vi "Entrenamiento Fuerza 8.vi"(8 "error in (no error)":errorcluster) -> (0 "error out":errorcluster)   [LabVIEW 2014]
panel:
  in  "E/A":bool
  out "Tiempo Restante":string="15 : 58"
  out "Tiempo Transcurrido":string="04 : 01"
  in  "Reset":bool
  out "Hola":string="4"
  out "Cluster":T1={"Label"="Start", "Cuadriceps"=0, "Isquiotibiales"=0, "Gluteos"=0, "Abdomen"=0, "Lumbares"=0, "Dorsales"=0, "Trapecio"=0, "Pectorales"=35, "Biceps"=87, "Opcional"=0, "Tiempo"=20, "Impulso"=4, "Ruptura"=1, "Frecuencia"=80, "Profundidad"=200, "Ganancia"=0.1, "Master"=54, "Slider"=0}
  out "Master Ind":string="54%"
  in  "Master":bool
  out "Master?":bool
  out "error out 2":errorcluster={"status"=FALSE, "code"=1073676418, "source"="VISA Close in Entrenamiento Fuerza 6.vi"}
  in  "Puerto Serial":refnum<visa-resource-name>="COM25"
  out "Start?":bool
  in  "Start":bool
  in  "Impulso":bool
  in  "Back":bool
  in  "Help":bool
  in  "Slider":i32(slide) scale=0.0..100.0
  out "Horizontal Graduated Bar":i16(slide) scale=0.0..100.0
  in  "Remove Button":bool
  in  "Add Button":bool
  out "Opcional %":string="0%"
  in  "Opcional Bool":bool
  out "Biceps %":string="87%"
  in  "Biceps Bool":bool
  out "Pectorales %":string="35%"
  in  "Pectorales Bool":bool
  out "Trapecio %":string="0%"
  in  "Trapecio Bool":bool
  out "Dorsales %":string="0%"
  in  "Dorsales Bool":bool
  out "Lumbares %":string="0%"
  in  "Lumbares Bool":bool
  out "Abdomen %":string="0%"
  in  "Abdomen Bool":bool
  out "Gluteos %":string="0%"
  in  "Gluteos Bool":bool
  out "Isquiotibiales %":string="0%"
  in  "Isquiotibiales Bool":bool
  out "Cuadríceps %":string="0%"
  in  "Cuadriceps Bool":bool
  out "date/time string":string="26/11/2015 06:09:03 p. m."
  # "Entrenamiento de Fuerza"
  # "Presentación"
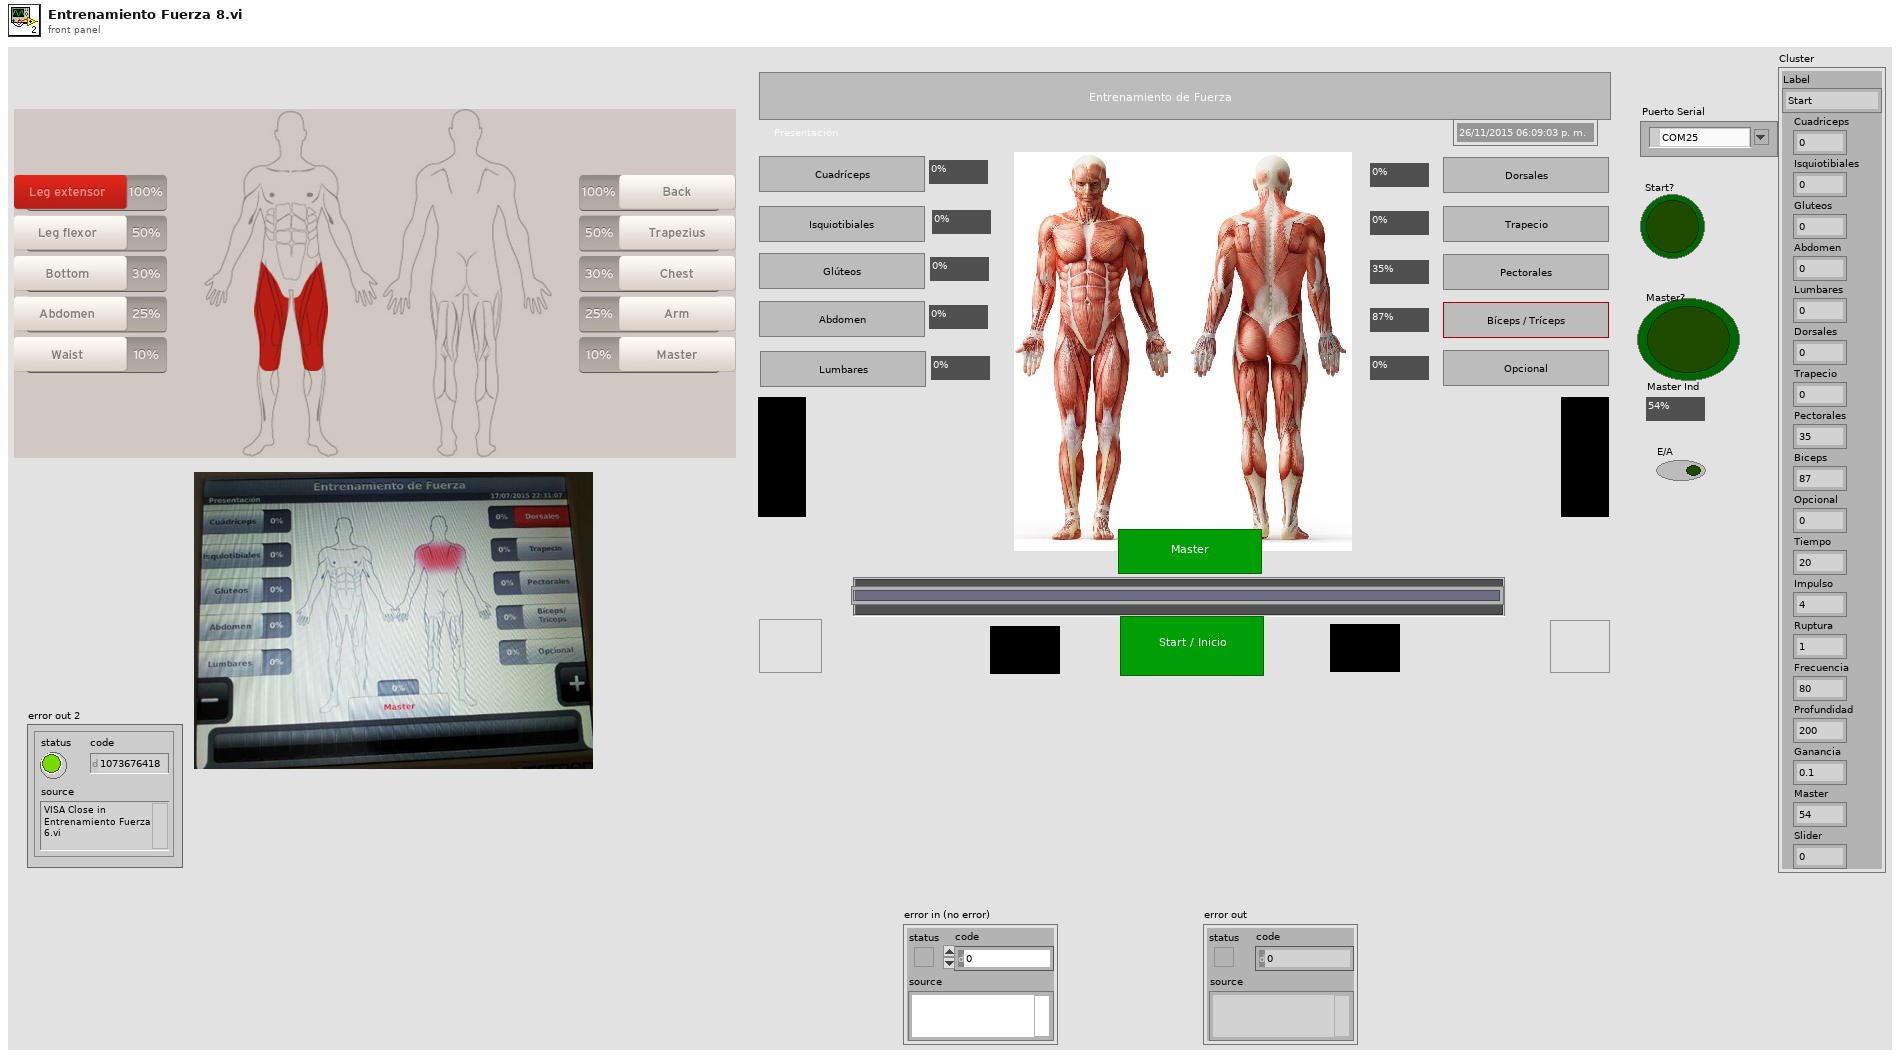
[diagram p1: front panel]
types:
  T1 = cluster{"Label":string, "Cuadriceps":i32, "Isquiotibiales":i32, "Gluteos":i32, "Abdomen":i32, "Lumbares":i32, "Dorsales":i32, "Trapecio":i32, "Pectorales":i32, "Biceps":i32, "Opcional":i32, "Tiempo":i32, "Impulso":i32, "Ruptura":i32, "Frecuencia":i32, "Profundidad":i32, "Ganancia":dbl, "Master":i32, "Slider":i32}
  T2 = cluster{"Label":string, "Cuadriceps":i32, "Isquiotibiales":i32, "Gluteos":i32, "Abdomen":i32, "Lumbares":i32, "Dorsales":i32, "Trapecio":i32, "Pectorales":i32, "Biceps":i32, "Opcional":i32, "Tiempo":i32, "Impulso":i32, "Ruptura":i32, "Frecuencia":i32, "Profundidad":i32, "Ganancia":i32, "Master":i32, "Slider":i32}
  T3 = cluster{u32, "Boolean Text.Text Colors:Text Color":u32}
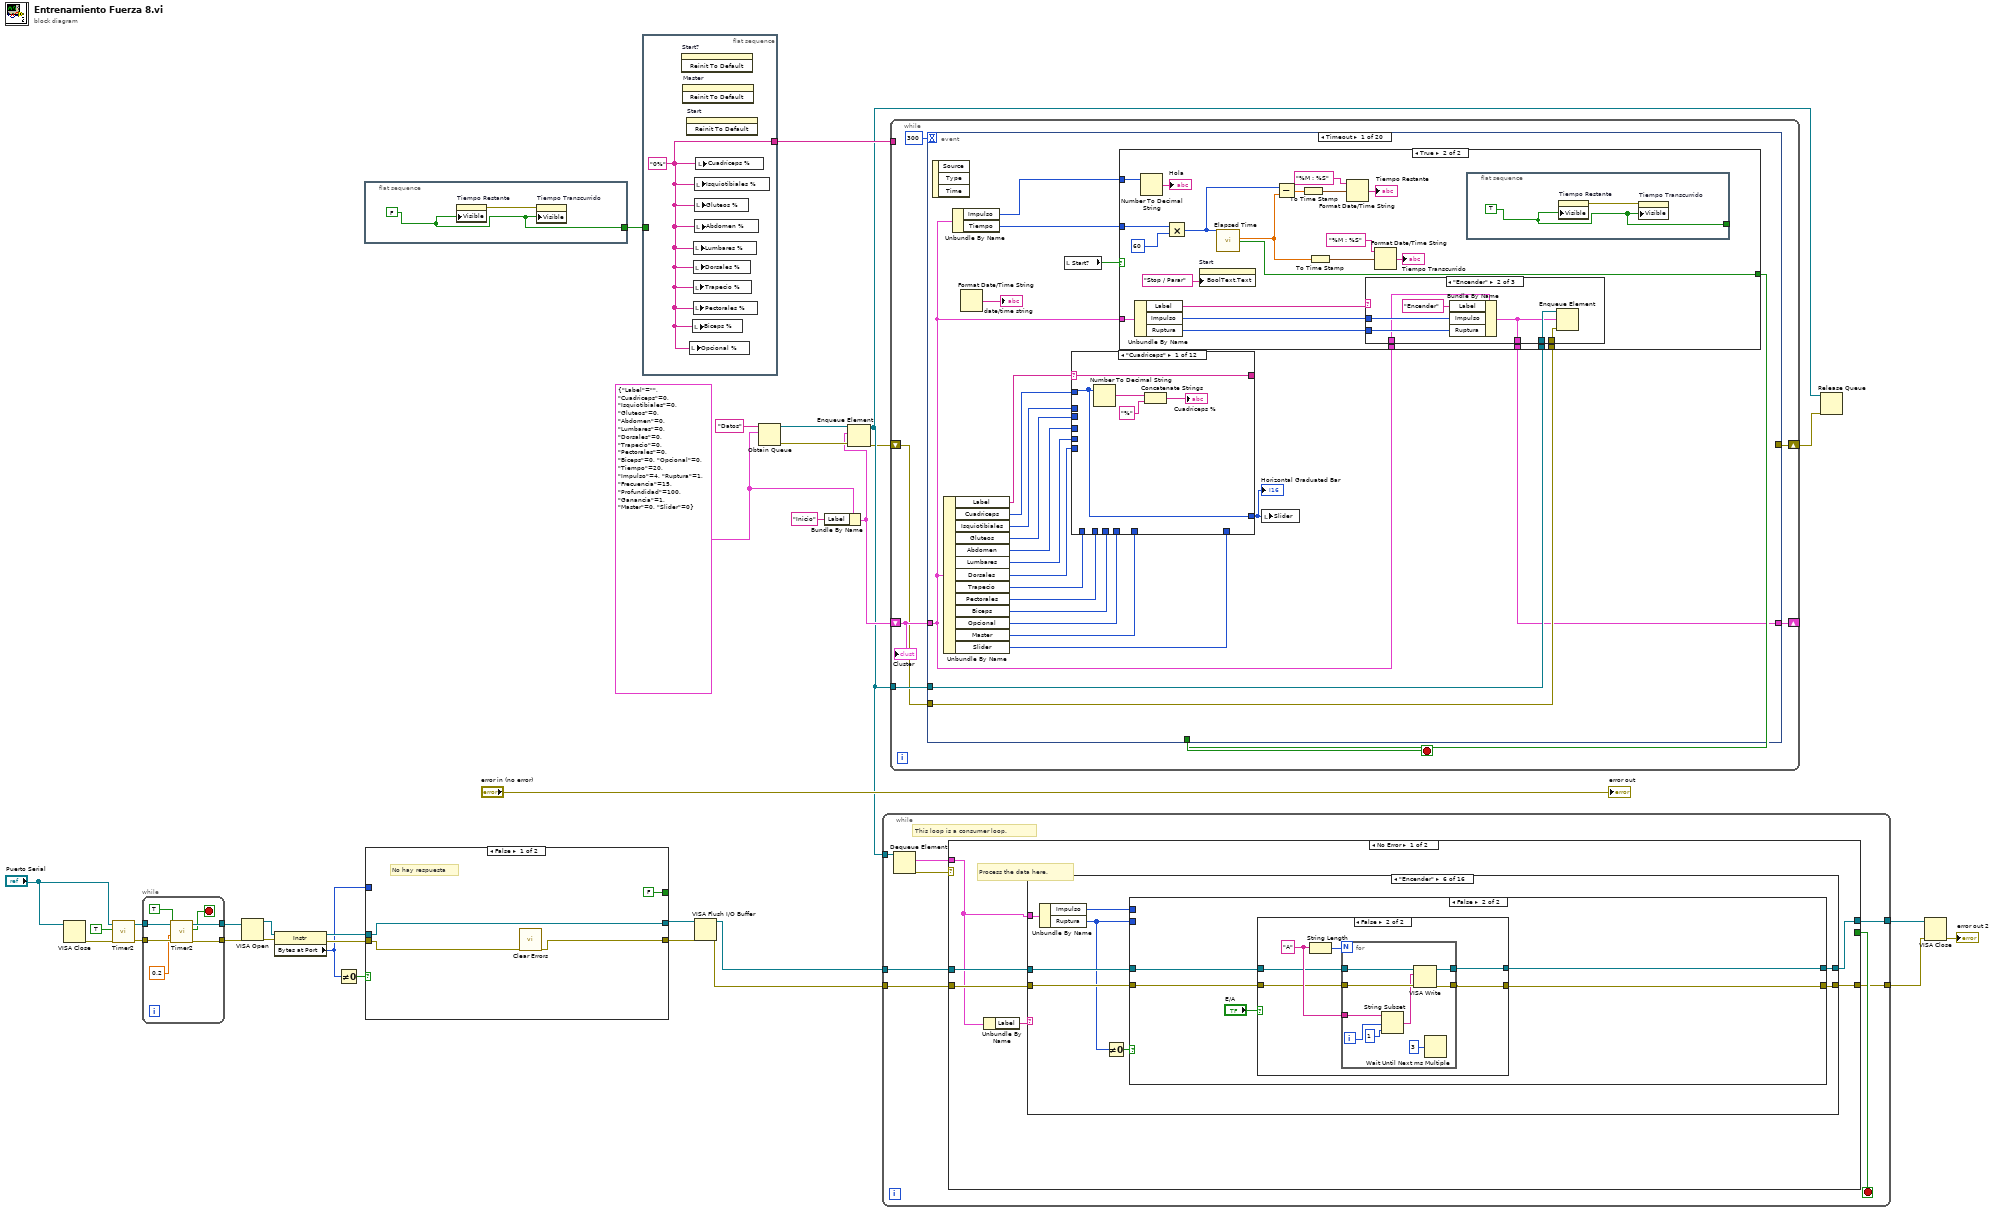
[diagram p0: block diagram]
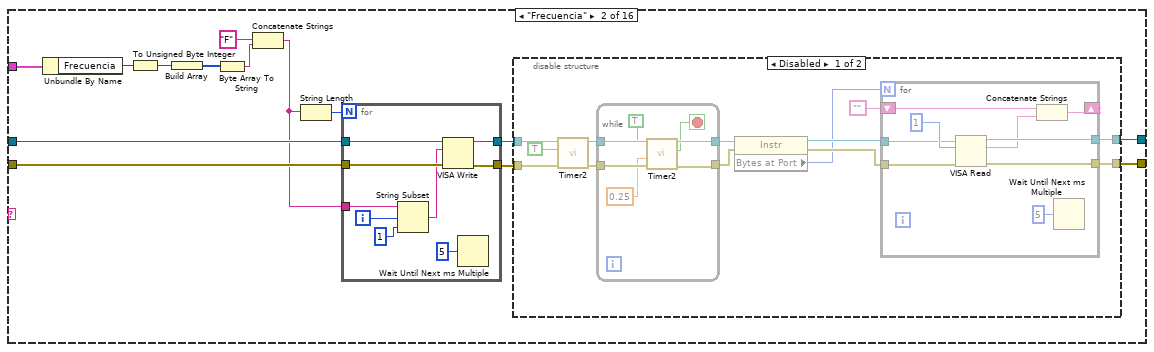
[diagram p3: hidden frame]
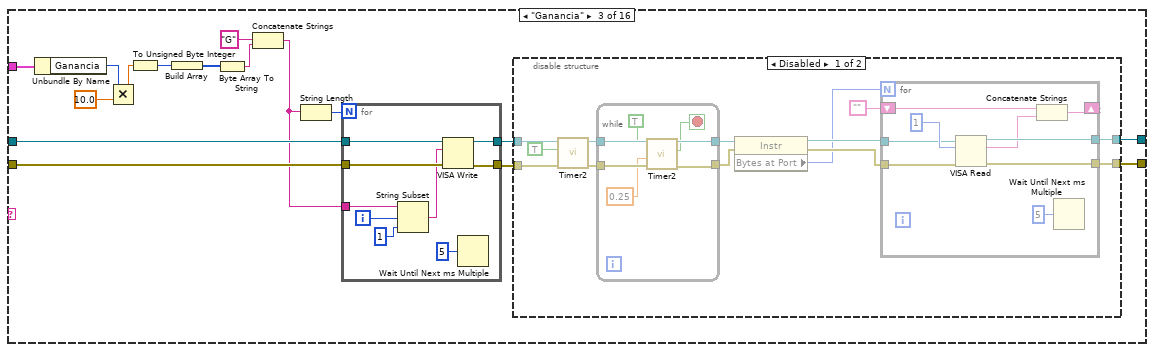
[diagram p5: hidden frame]
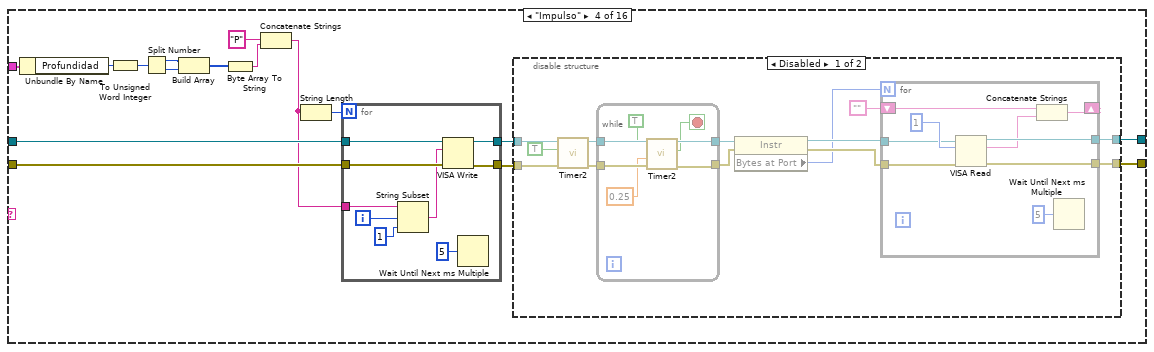
[diagram p7: hidden frame]
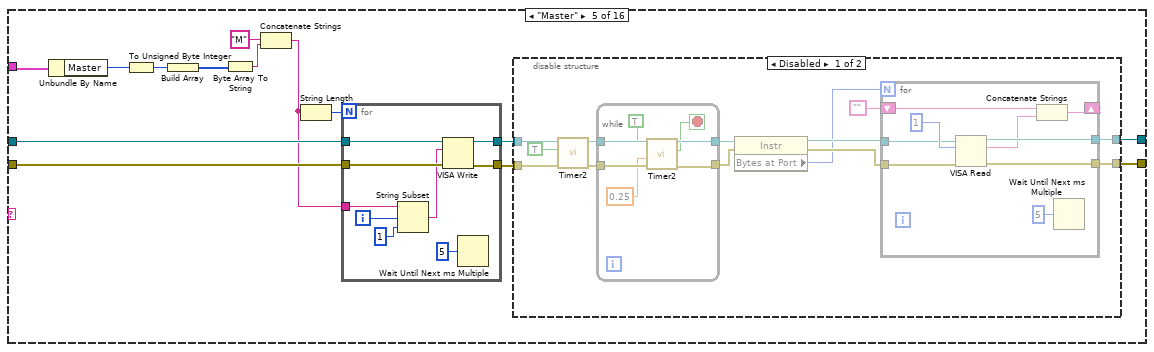
[diagram p9: hidden frame]
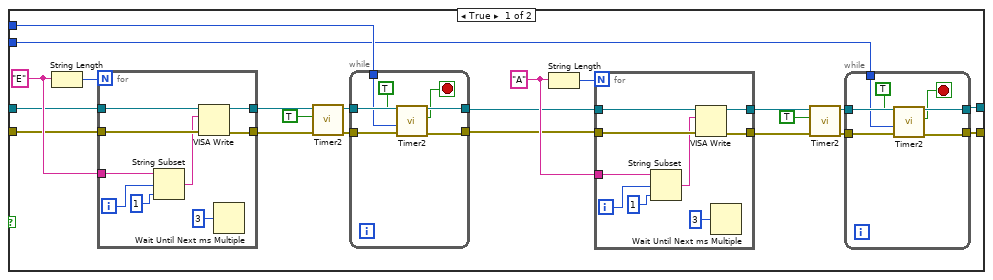
[diagram p11: hidden frame]
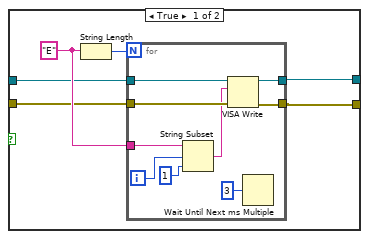
[diagram p12: hidden frame]
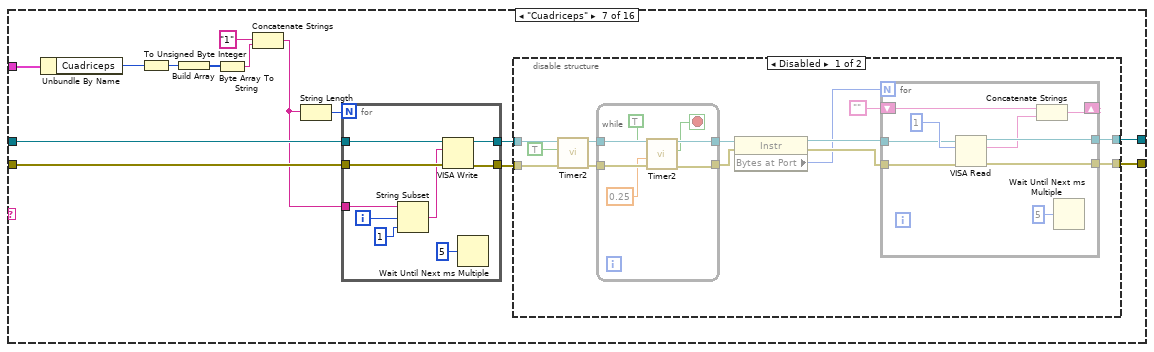
[diagram p13: hidden frame]
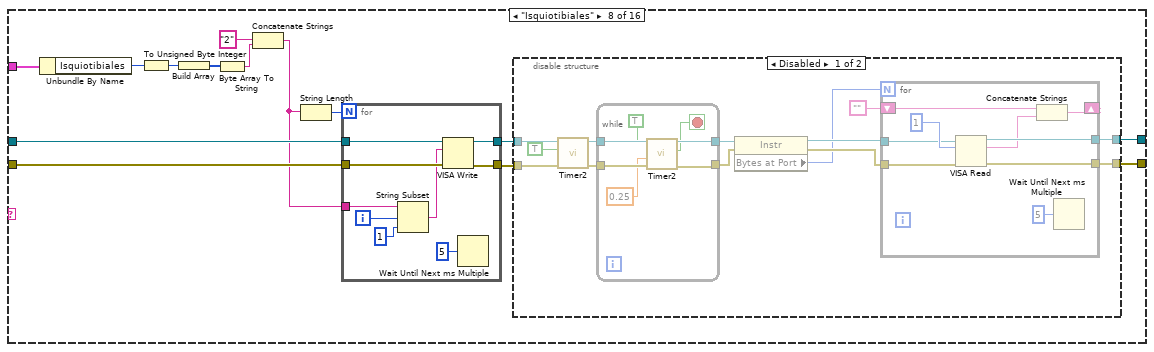
[diagram p15: hidden frame]
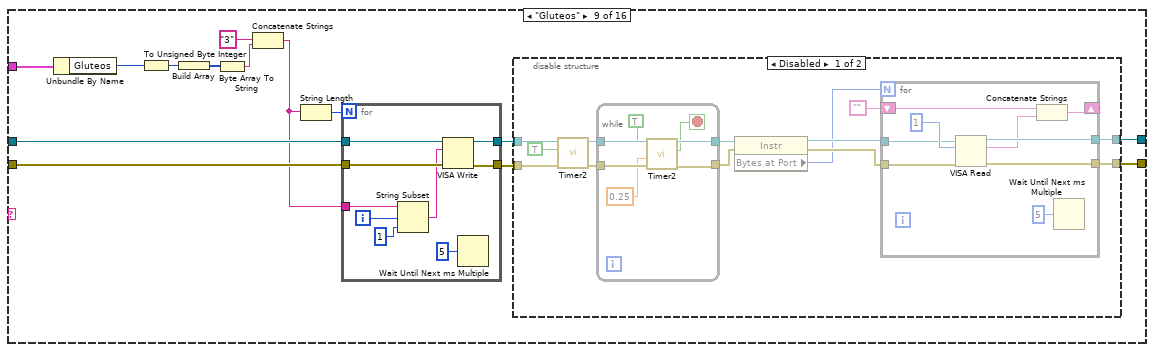
[diagram p17: hidden frame]
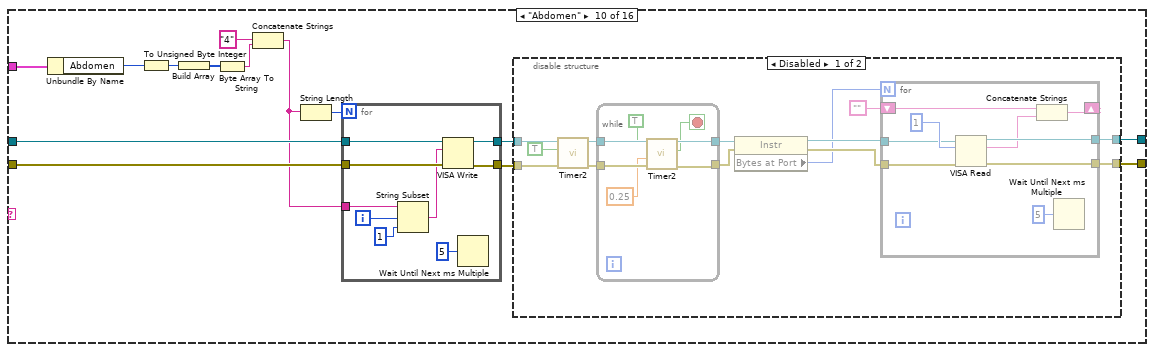
[diagram p19: hidden frame]
diagram:
  w12 = T2 {"Label"="", "Cuadriceps"=0, "Isquiotibiales"=0, "Gluteos"=0, "Abdomen"=0, "Lumbares"=0, "Dorsales"=0, "Trapecio"=0, "Pectorales"=0, "Biceps"=0, "Opcional"=0, "Tiempo"=20, "Impulso"=4, "Ruptura"=1, "Frecuencia"=15, "Profundidad"=100, "Ganancia"=1, "Master"=0, "Slider"=0}
  n1 = VISA Close(VISA resource name="Puerto Serial") -> (error out=w27:errorcluster)  [unwired: 1 in]
  n2 = call "Timer2.vi"("error in (no error)"=w27, "Reset"=TRUE) -> ("error out"=w26:errorcluster)  [unwired: 7 in, 2 out]
  n3 = while {
    tunnel: w26 -> [w36]
    tunnel: "Puerto Serial" -> [w37]
    tunnel: [w37] -> w28
    tunnel: [w35] -> w24
    stop <- w34 stop-if-true
    n4 = call "Timer2.vi"("error in (no error)"=w36, "Time Target (s)"=0.2, "Pause"=TRUE) -> ("error out"=w35:errorcluster, "Time has Elapsed"=w34:bool)  [unwired: 6 in, 1 out]
  }
  n5 = VISA Open(error in (no error)=w24, VISA resource name=w28) -> (VISA resource name=w16:refnum<visa-resource-name>, error out=w17:errorcluster)  [unwired: 3 in]
  n6 = property class="Instr"(reference=w16, error in=w17) -> (reference out=w22:refnum<visa-resource-name>, error out=w23:errorcluster, "Bytes at Port"=w20:u32)
  n7 = Not Equal To 0?(x=w20) -> (x != 0?=w21:bool)
  n8 = flat-sequence {
    tunnel: [w38] -> w1
    frame #0 {
      w38 = FALSE ("Visible")
      n9 = property on="Tiempo Restante" class="Str"("Visible"=w38) -> (error out=w39:errorcluster)  [unwired: 2 in, 1 out]
      n10 = property on="Tiempo Transcurrido" class="Str"(error in=w39, "Visible"=w38) -> ()  [unwired: 1 in, 2 out]
    }
  }
  n11 = case shown="False" w21 {
    tunnel: w23 -> [w41 w51]
    tunnel: w22 -> [w43 w50]
    tunnel: w20 -> [_ w49]
    tunnel: [w43 w47] -> w18
    tunnel: [w40 w46] -> w19
    tunnel: [FALSE w45] -> _
    frame False {
      # "No hay respuesta"
      n12 = call <vilib>:"Clear Errors.vi"("error in (no error)"=w41) -> ("error out"=w40:errorcluster)  [unwired: 5 in, 1 out]
    }
    frame True {
      # "Recibe Datos de Respuesta"
      n13 = for {
        N: w49 -> [_]
        tunnel: w51 -> [w60]
        tunnel: w50 -> [w59]
        shift-right: [w54] -> w44
        shift-left: "" -> [w58]
        tunnel: [w57] -> w46
        tunnel: [w56] -> w47
        n14 = VISA Read(VISA resource name=w59, byte count=u32 1, error in (no error)=w60) -> (VISA resource name out=w56:refnum<visa-resource-name>, read buffer=w53:string, error out=w57:errorcluster)  [unwired: 1 out]
        n15 = Concatenate Strings(w58, w53) -> (w54:string)
        n16 = Wait Until Next ms Multiple(millisecond multiple=u32 1) -> ()  [unwired: 1 out]
      }
      n17 = Equal?(x=w44, y="OK") -> (x = y?=w45:bool)
    }
  }
  n18 = flat-sequence {
    tunnel: [w62] -> w15
    tunnel: w1 -> [_]
    frame #0 {
      w62 = "0%" ("Cuadríceps %")
      n19 = invoke on="Start?" class="Bool (strict)" method="Reinit To Default"() -> ()  [unwired: 3 in, 3 out]
      n20 = invoke on="Master" class="Bool (strict)" method="Reinit To Default"() -> ()  [unwired: 3 in, 3 out]
      n21 = invoke on="Start" class="Bool (strict)" method="Reinit To Default"() -> ()  [unwired: 3 in, 3 out]
      n22 = local write "Opcional %"(w62) -> ()
      n23 = local write "Biceps %"(w62) -> ()
      n24 = local write "Trapecio %"(w62) -> ()
      n25 = local write "Pectorales %"(w62) -> ()
      n26 = local write "Lumbares %"(w62) -> ()
      n27 = local write "Dorsales %"(w62) -> ()
      n28 = local write "Isquiotibiales %"(w62) -> ()
      n29 = local write "Gluteos %"(w62) -> ()
      n30 = local write "Abdomen %"(w62) -> ()
      n31 = local write "Cuadríceps %"(w62) -> ()
    }
  }
  n32 = VISA Flush I/O Buffer(VISA resource name=w18, error in (no error)=w19) -> (VISA resource name out=w7:refnum<visa-resource-name>, error out=w6:errorcluster)  [unwired: 1 in]
  n33 = Obtain Queue(name (unnamed)="Datos", element data type=w12) -> (queue out=w13:refnum<queue>, error out=w14:errorcluster)  [unwired: 3 in, 1 out]
  n34 = Bundle By Name(cluster=w12, "Label"="Inicio") -> (w10:T2)
  n35 = Enqueue Element(queue=w13, element=w10, error in (no error)=w14) -> (queue out=w8:refnum<queue>, error out=w3:errorcluster)  [unwired: 1 in, 1 out]
  n36 = while {
    tunnel: w8 -> [w70]
    tunnel: w7 -> [w66]
    tunnel: w6 -> [w65]
    tunnel: [w64] -> w5
    tunnel: [w63] -> w4
    stop <- w67 stop-if-true
    # "This loop is a consumer loop."
    n37 = Dequeue Element(queue=w70) -> (element=w68:T2, error out=w69:errorcluster)  [unwired: 2 in, 2 out]
    n38 = case shown="No Error" w69 {
      tunnel: w68 -> [w71 _]
      tunnel: [_ TRUE] -> w67
      tunnel: w66 -> [w76 w904]
      tunnel: w65 -> [w75 w905]
      tunnel: [w74 w904] -> w64
      tunnel: [w73 w905] -> w63
      frame No Error {
        # "Process the data here."
        n39 = Unbundle By Name(w71) -> ("Label"=w72:string)
        n40 = case shown="\"Encender\"" w72 {
          tunnel: w76 -> [w77 w92 w146 w200 w252 w295 w397 w449 w501 w553 w605 w657 w709 w761 w813 w865]
          tunnel: w75 -> [w78 w91 w145 w199 w251 w294 w396 w448 w500 w552 w604 w656 w708 w760 w812 w864]
          tunnel: [w78 w90 w144 w198 w250 w297 w395 w447 w499 w551 w603 w655 w707 w759 w811 w863] -> w73
          tunnel: [w77 w89 w143 w197 w249 w296 w394 w446 w498 w550 w602 w654 w706 w758 w810 w862] -> w74
          tunnel: w71 -> [_ w81 w136 w190 w239 w298 w386 w438 w490 w542 w594 w646 w698 w750 w802 w854]
          frame "Inicio", Default {
          }
          frame "Frecuencia" {
            n41 = Unbundle By Name(w81) -> ("Frecuencia"=w82:i32)
            n42 = To Unsigned Byte Integer(number=w82) -> (unsigned 8bit integer=w80:u8)
            n43 = Build Array(w80) -> (w79:u8[])
            n44 = Byte Array To String(unsigned byte array=w79) -> (string=w84:string)
            n45 = Concatenate Strings("F", w84) -> (w83:string)
            n46 = String Length(string=w83) -> (length=w88:i32)
            n47 = for {
              N: w88 -> [_]
              tunnel: w91 -> [w130]
              tunnel: w92 -> [w129]
              tunnel: w83 -> [w126]
              tunnel: [w123] -> w86
              tunnel: [w122] -> w87
              i -> [w124]
              n48 = String Subset(string=w126, offset (0)=w124, length (rest)=1 ("length (rest)")) -> (substring=w127:string)
              n49 = VISA Write(VISA resource name=w129, write buffer=w127, error in (no error)=w130) -> (VISA resource name out=w122:refnum<visa-resource-name>, error out=w123:errorcluster)  [unwired: 1 out]
              n50 = Wait Until Next ms Multiple(millisecond multiple=u32 5) -> ()  [unwired: 1 out]
            }
            n51 = disable-structure shown="Disabled" {
              disable-tunnel: [w104 w120] -> w90
              disable-tunnel: [w103 w121] -> w89
              disable-tunnel: w87 -> [w98 w121]
              disable-tunnel: w86 -> [w94 w120]
              frame Disabled {
                n52 = call "Timer2.vi"("error in (no error)"=w94, "Reset"=TRUE) -> ("error out"=w93:errorcluster)  [unwired: 7 in, 2 out]
                n53 = while {
                  tunnel: w98 -> [w110]
                  tunnel: [w110] -> w97
                  tunnel: [w108] -> w96
                  tunnel: w93 -> [w109]
                  stop <- w107 stop-if-true
                  n54 = call "Timer2.vi"("error in (no error)"=w109, "Time Target (s)"=0.25, "Pause"=TRUE) -> ("error out"=w108:errorcluster, "Time has Elapsed"=w107:bool)  [unwired: 6 in, 1 out]
                }
                n55 = property class="Instr"(reference=w97, error in=w96) -> (reference out=w101:refnum<visa-resource-name>, error out=w100:errorcluster, "Bytes at Port"=w99:u32)
                n56 = for {
                  N: w99 -> [_]
                  tunnel: w100 -> [w118]
                  tunnel: w101 -> [w117]
                  shift-right: [w112] -> _
                  shift-left: "" -> [w116]
                  tunnel: [w115] -> w104
                  tunnel: [w114] -> w103
                  n57 = VISA Read(VISA resource name=w117, byte count=u32 1, error in (no error)=w118) -> (VISA resource name out=w114:refnum<visa-resource-name>, read buffer=w111:string, error out=w115:errorcluster)  [unwired: 1 out]
                  n58 = Concatenate Strings(w116, w111) -> (w112:string)
                  n59 = Wait Until Next ms Multiple(millisecond multiple=u32 5) -> ()  [unwired: 1 out]
                }
              }
              frame Enabled {
              }
            }
          }
          frame "Ganancia" {
            n60 = Unbundle By Name(w136) -> ("Ganancia"=w132:i32)
            n61 = Multiply(x=w132, y=10.0) -> (x*y=w133:dbl)
            n62 = To Unsigned Byte Integer(number=w133) -> (unsigned 8bit integer=w135:u8)
            n63 = Build Array(w135) -> (w134:u8[])
            n64 = Byte Array To String(unsigned byte array=w134) -> (string=w138:string)
            n65 = Concatenate Strings("G", w138) -> (w137:string)
            n66 = String Length(string=w137) -> (length=w142:i32)
            n67 = for {
              N: w142 -> [_]
              tunnel: w145 -> [w184]
              tunnel: w146 -> [w183]
              tunnel: w137 -> [w180]
              tunnel: [w177] -> w140
              tunnel: [w176] -> w141
              i -> [w178]
              n68 = String Subset(string=w180, offset (0)=w178, length (rest)=1 ("length (rest)")) -> (substring=w181:string)
              n69 = VISA Write(VISA resource name=w183, write buffer=w181, error in (no error)=w184) -> (VISA resource name out=w176:refnum<visa-resource-name>, error out=w177:errorcluster)  [unwired: 1 out]
              n70 = Wait Until Next ms Multiple(millisecond multiple=u32 5) -> ()  [unwired: 1 out]
            }
            n71 = disable-structure shown="Disabled" {
              disable-tunnel: [w158 w174] -> w144
              disable-tunnel: [w157 w175] -> w143
              disable-tunnel: w141 -> [w152 w175]
              disable-tunnel: w140 -> [w148 w174]
              frame Disabled {
                n72 = call "Timer2.vi"("error in (no error)"=w148, "Reset"=TRUE) -> ("error out"=w147:errorcluster)  [unwired: 7 in, 2 out]
                n73 = while {
                  tunnel: w152 -> [w164]
                  tunnel: [w164] -> w151
                  tunnel: [w162] -> w150
                  tunnel: w147 -> [w163]
                  stop <- w161 stop-if-true
                  n74 = call "Timer2.vi"("error in (no error)"=w163, "Time Target (s)"=0.25, "Pause"=TRUE) -> ("error out"=w162:errorcluster, "Time has Elapsed"=w161:bool)  [unwired: 6 in, 1 out]
                }
                n75 = property class="Instr"(reference=w151, error in=w150) -> (reference out=w155:refnum<visa-resource-name>, error out=w154:errorcluster, "Bytes at Port"=w153:u32)
                n76 = for {
                  N: w153 -> [_]
                  tunnel: w154 -> [w172]
                  tunnel: w155 -> [w171]
                  shift-right: [w166] -> _
                  shift-left: "" -> [w170]
                  tunnel: [w169] -> w158
                  tunnel: [w168] -> w157
                  n77 = VISA Read(VISA resource name=w171, byte count=u32 1, error in (no error)=w172) -> (VISA resource name out=w168:refnum<visa-resource-name>, read buffer=w165:string, error out=w169:errorcluster)  [unwired: 1 out]
                  n78 = Concatenate Strings(w170, w165) -> (w166:string)
                  n79 = Wait Until Next ms Multiple(millisecond multiple=u32 5) -> ()  [unwired: 1 out]
                }
              }
              frame Enabled {
              }
            }
          }
          frame "Impulso" {
            n80 = Unbundle By Name(w190) -> ("Profundidad"=w187:i32)
            n81 = To Unsigned Word Integer(number=w187) -> (unsigned 16bit integer=w186:u16)
            n82 = Split Number(x=w186) -> (hi(x)=w189:u8, lo(x)=w188:u8)
            n83 = Build Array(w189, w188) -> (w185:u8[])
            n84 = Byte Array To String(unsigned byte array=w185) -> (string=w192:string)
            n85 = Concatenate Strings("P", w192) -> (w191:string)
            n86 = String Length(string=w191) -> (length=w196:i32)
            n87 = for {
              N: w196 -> [_]
              tunnel: w199 -> [w238]
              tunnel: w200 -> [w237]
              tunnel: w191 -> [w234]
              tunnel: [w231] -> w194
              tunnel: [w230] -> w195
              i -> [w232]
              n88 = String Subset(string=w234, offset (0)=w232, length (rest)=1 ("length (rest)")) -> (substring=w235:string)
              n89 = VISA Write(VISA resource name=w237, write buffer=w235, error in (no error)=w238) -> (VISA resource name out=w230:refnum<visa-resource-name>, error out=w231:errorcluster)  [unwired: 1 out]
              n90 = Wait Until Next ms Multiple(millisecond multiple=u32 5) -> ()  [unwired: 1 out]
            }
            n91 = disable-structure shown="Disabled" {
              disable-tunnel: [w212 w228] -> w198
              disable-tunnel: [w211 w229] -> w197
              disable-tunnel: w195 -> [w206 w229]
              disable-tunnel: w194 -> [w202 w228]
              frame Disabled {
                n92 = call "Timer2.vi"("error in (no error)"=w202, "Reset"=TRUE) -> ("error out"=w201:errorcluster)  [unwired: 7 in, 2 out]
                n93 = while {
                  tunnel: w206 -> [w218]
                  tunnel: [w218] -> w205
                  tunnel: [w216] -> w204
                  tunnel: w201 -> [w217]
                  stop <- w215 stop-if-true
                  n94 = call "Timer2.vi"("error in (no error)"=w217, "Time Target (s)"=0.25, "Pause"=TRUE) -> ("error out"=w216:errorcluster, "Time has Elapsed"=w215:bool)  [unwired: 6 in, 1 out]
                }
                n95 = property class="Instr"(reference=w205, error in=w204) -> (reference out=w209:refnum<visa-resource-name>, error out=w208:errorcluster, "Bytes at Port"=w207:u32)
                n96 = for {
                  N: w207 -> [_]
                  tunnel: w208 -> [w226]
                  tunnel: w209 -> [w225]
                  shift-right: [w220] -> _
                  shift-left: "" -> [w224]
                  tunnel: [w223] -> w212
                  tunnel: [w222] -> w211
                  n97 = VISA Read(VISA resource name=w225, byte count=u32 1, error in (no error)=w226) -> (VISA resource name out=w222:refnum<visa-resource-name>, read buffer=w219:string, error out=w223:errorcluster)  [unwired: 1 out]
                  n98 = Concatenate Strings(w224, w219) -> (w220:string)
                  n99 = Wait Until Next ms Multiple(millisecond multiple=u32 5) -> ()  [unwired: 1 out]
                }
              }
              frame Enabled {
              }
            }
          }
          frame "Master" {
            n100 = Unbundle By Name(w239) -> ("Master"=w242:i32)
            n101 = To Unsigned Byte Integer(number=w242) -> (unsigned 8bit integer=w241:u8)
            n102 = Build Array(w241) -> (w240:u8[])
            n103 = Byte Array To String(unsigned byte array=w240) -> (string=w244:string)
            n104 = Concatenate Strings("M", w244) -> (w243:string)
            n105 = String Length(string=w243) -> (length=w248:i32)
            n106 = for {
              N: w248 -> [_]
              tunnel: w251 -> [w290]
              tunnel: w252 -> [w289]
              tunnel: w243 -> [w286]
              tunnel: [w283] -> w246
              tunnel: [w282] -> w247
              i -> [w284]
              n107 = String Subset(string=w286, offset (0)=w284, length (rest)=1 ("length (rest)")) -> (substring=w287:string)
              n108 = VISA Write(VISA resource name=w289, write buffer=w287, error in (no error)=w290) -> (VISA resource name out=w282:refnum<visa-resource-name>, error out=w283:errorcluster)  [unwired: 1 out]
              n109 = Wait Until Next ms Multiple(millisecond multiple=u32 5) -> ()  [unwired: 1 out]
            }
            n110 = disable-structure shown="Disabled" {
              disable-tunnel: [w264 w280] -> w250
              disable-tunnel: [w263 w281] -> w249
              disable-tunnel: w247 -> [w258 w281]
              disable-tunnel: w246 -> [w254 w280]
              frame Disabled {
                n111 = call "Timer2.vi"("error in (no error)"=w254, "Reset"=TRUE) -> ("error out"=w253:errorcluster)  [unwired: 7 in, 2 out]
                n112 = while {
                  tunnel: w258 -> [w270]
                  tunnel: [w270] -> w257
                  tunnel: [w268] -> w256
                  tunnel: w253 -> [w269]
                  stop <- w267 stop-if-true
                  n113 = call "Timer2.vi"("error in (no error)"=w269, "Time Target (s)"=0.25, "Pause"=TRUE) -> ("error out"=w268:errorcluster, "Time has Elapsed"=w267:bool)  [unwired: 6 in, 1 out]
                }
                n114 = property class="Instr"(reference=w257, error in=w256) -> (reference out=w261:refnum<visa-resource-name>, error out=w260:errorcluster, "Bytes at Port"=w259:u32)
                n115 = for {
                  N: w259 -> [_]
                  tunnel: w260 -> [w278]
                  tunnel: w261 -> [w277]
                  shift-right: [w272] -> _
                  shift-left: "" -> [w276]
                  tunnel: [w275] -> w264
                  tunnel: [w274] -> w263
                  n116 = VISA Read(VISA resource name=w277, byte count=u32 1, error in (no error)=w278) -> (VISA resource name out=w274:refnum<visa-resource-name>, read buffer=w271:string, error out=w275:errorcluster)  [unwired: 1 out]
                  n117 = Concatenate Strings(w276, w271) -> (w272:string)
                  n118 = Wait Until Next ms Multiple(millisecond multiple=u32 5) -> ()  [unwired: 1 out]
                }
              }
              frame Enabled {
              }
            }
          }
          frame "Encender" {
            n119 = Unbundle By Name(w298) -> ("Impulso"=w293:i32, "Ruptura"=w291:i32)
            n120 = Not Equal To 0?(x=w291) -> (x != 0?=w292:bool)
            n121 = case shown="False" w292 {
              tunnel: [w304 w351] -> w297
              tunnel: [w303 w350] -> w296
              tunnel: w295 -> [w302 w353]
              tunnel: w294 -> [w301 w352]
              tunnel: w293 -> [w300 _]
              tunnel: w291 -> [w299 _]
              frame True {
                w309 = "A"
                w315 = "E"
                n122 = String Length(string=w315) -> (length=w318:i32)
                n123 = for {
                  N: w318 -> [_]
                  tunnel: w301 -> [w348]
                  tunnel: w302 -> [w347]
                  tunnel: w315 -> [w344]
                  tunnel: [w341] -> w316
                  tunnel: [w340] -> w317
                  i -> [w342]
                  n124 = String Subset(string=w344, offset (0)=w342, length (rest)=1 ("length (rest)")) -> (substring=w345:string)
                  n125 = VISA Write(VISA resource name=w347, write buffer=w345, error in (no error)=w348) -> (VISA resource name out=w340:refnum<visa-resource-name>, error out=w341:errorcluster)  [unwired: 1 out]
                  n126 = Wait Until Next ms Multiple(millisecond multiple=u32 3) -> ()  [unwired: 1 out]
                }
                n127 = call "Timer2.vi"("error in (no error)"=w316, "Reset"=TRUE) -> ("error out"=w313:errorcluster)  [unwired: 7 in, 2 out]
                n128 = while {
                  tunnel: w317 -> [w339]
                  tunnel: [w339] -> w306
                  tunnel: [w337] -> w305
                  tunnel: w313 -> [w338]
                  tunnel: w300 -> [w334]
                  stop <- w336 stop-if-true
                  n129 = call "Timer2.vi"("error in (no error)"=w338, "Time Target (s)"=w334, "Pause"=TRUE) -> ("error out"=w337:errorcluster, "Time has Elapsed"=w336:bool)  [unwired: 6 in, 1 out]
                }
                n130 = String Length(string=w309) -> (length=w312:i32)
                n131 = for {
                  N: w312 -> [_]
                  tunnel: w305 -> [w333]
                  tunnel: w306 -> [w332]
                  tunnel: w309 -> [w329]
                  tunnel: [w326] -> w310
                  tunnel: [w325] -> w311
                  i -> [w327]
                  n132 = String Subset(string=w329, offset (0)=w327, length (rest)=1 ("length (rest)")) -> (substring=w330:string)
                  n133 = VISA Write(VISA resource name=w332, write buffer=w330, error in (no error)=w333) -> (VISA resource name out=w325:refnum<visa-resource-name>, error out=w326:errorcluster)  [unwired: 1 out]
                  n134 = Wait Until Next ms Multiple(millisecond multiple=u32 3) -> ()  [unwired: 1 out]
                }
                n135 = call "Timer2.vi"("error in (no error)"=w310, "Reset"=TRUE) -> ("error out"=w307:errorcluster)  [unwired: 7 in, 2 out]
                n136 = while {
                  tunnel: w311 -> [w324]
                  tunnel: [w324] -> w303
                  tunnel: [w322] -> w304
                  tunnel: w307 -> [w323]
                  tunnel: w299 -> [w319]
                  stop <- w321 stop-if-true
                  n137 = call "Timer2.vi"("error in (no error)"=w323, "Time Target (s)"=w319, "Pause"=TRUE) -> ("error out"=w322:errorcluster, "Time has Elapsed"=w321:bool)  [unwired: 6 in, 1 out]
                }
              }
              frame False {
                n138 = case shown="False" "E/A" {
                  tunnel: w353 -> [w357 w372]
                  tunnel: w352 -> [w356 w371]
                  tunnel: [w355 w370] -> w351
                  tunnel: [w354 w369] -> w350
                  frame True {
                    w358 = "E"
                    n139 = String Length(string=w358) -> (length=w359:i32)
                    n140 = for {
                      N: w359 -> [_]
                      tunnel: w356 -> [w368]
                      tunnel: w357 -> [w367]
                      tunnel: w358 -> [w364]
                      tunnel: [w361] -> w355
                      tunnel: [w360] -> w354
                      i -> [w362]
                      n141 = String Subset(string=w364, offset (0)=w362, length (rest)=1 ("length (rest)")) -> (substring=w365:string)
                      n142 = VISA Write(VISA resource name=w367, write buffer=w365, error in (no error)=w368) -> (VISA resource name out=w360:refnum<visa-resource-name>, error out=w361:errorcluster)  [unwired: 1 out]
                      n143 = Wait Until Next ms Multiple(millisecond multiple=u32 3) -> ()  [unwired: 1 out]
                    }
                  }
                  frame False {
                    w373 = "A"
                    n144 = String Length(string=w373) -> (length=w374:i32)
                    n145 = for {
                      N: w374 -> [_]
                      tunnel: w371 -> [w383]
                      tunnel: w372 -> [w382]
                      tunnel: w373 -> [w379]
                      tunnel: [w376] -> w370
                      tunnel: [w375] -> w369
                      i -> [w377]
                      n146 = String Subset(string=w379, offset (0)=w377, length (rest)=1 ("length (rest)")) -> (substring=w380:string)
                      n147 = VISA Write(VISA resource name=w382, write buffer=w380, error in (no error)=w383) -> (VISA resource name out=w375:refnum<visa-resource-name>, error out=w376:errorcluster)  [unwired: 1 out]
                      n148 = Wait Until Next ms Multiple(millisecond multiple=u32 3) -> ()  [unwired: 1 out]
                    }
                  }
                }
              }
            }
          }
          frame "Cuadriceps" {
            n149 = Unbundle By Name(w386) -> ("Cuadriceps"=w384:i32)
            n150 = To Unsigned Byte Integer(number=w384) -> (unsigned 8bit integer=w385:u8)
            n151 = Build Array(w385) -> (w390:u8[])
            n152 = Byte Array To String(unsigned byte array=w390) -> (string=w388:string)
            n153 = Concatenate Strings("1", w388) -> (w387:string)
            n154 = String Length(string=w387) -> (length=w393:i32)
            n155 = for {
              N: w393 -> [_]
              tunnel: w396 -> [w435]
              tunnel: w397 -> [w434]
              tunnel: w387 -> [w431]
              tunnel: [w428] -> w391
              tunnel: [w427] -> w392
              i -> [w429]
              n156 = String Subset(string=w431, offset (0)=w429, length (rest)=1 ("length (rest)")) -> (substring=w432:string)
              n157 = VISA Write(VISA resource name=w434, write buffer=w432, error in (no error)=w435) -> (VISA resource name out=w427:refnum<visa-resource-name>, error out=w428:errorcluster)  [unwired: 1 out]
              n158 = Wait Until Next ms Multiple(millisecond multiple=u32 5) -> ()  [unwired: 1 out]
            }
            n159 = disable-structure shown="Disabled" {
              disable-tunnel: [w409 w425] -> w395
              disable-tunnel: [w408 w426] -> w394
              disable-tunnel: w392 -> [w403 w426]
              disable-tunnel: w391 -> [w399 w425]
              frame Disabled {
                n160 = call "Timer2.vi"("error in (no error)"=w399, "Reset"=TRUE) -> ("error out"=w398:errorcluster)  [unwired: 7 in, 2 out]
                n161 = while {
                  tunnel: w403 -> [w415]
                  tunnel: [w415] -> w402
                  tunnel: [w413] -> w401
                  tunnel: w398 -> [w414]
                  stop <- w412 stop-if-true
                  n162 = call "Timer2.vi"("error in (no error)"=w414, "Time Target (s)"=0.25, "Pause"=TRUE) -> ("error out"=w413:errorcluster, "Time has Elapsed"=w412:bool)  [unwired: 6 in, 1 out]
                }
                n163 = property class="Instr"(reference=w402, error in=w401) -> (reference out=w406:refnum<visa-resource-name>, error out=w405:errorcluster, "Bytes at Port"=w404:u32)
                n164 = for {
                  N: w404 -> [_]
                  tunnel: w405 -> [w423]
                  tunnel: w406 -> [w422]
                  shift-right: [w417] -> _
                  shift-left: "" -> [w421]
                  tunnel: [w420] -> w409
                  tunnel: [w419] -> w408
                  n165 = VISA Read(VISA resource name=w422, byte count=u32 1, error in (no error)=w423) -> (VISA resource name out=w419:refnum<visa-resource-name>, read buffer=w416:string, error out=w420:errorcluster)  [unwired: 1 out]
                  n166 = Concatenate Strings(w421, w416) -> (w417:string)
                  n167 = Wait Until Next ms Multiple(millisecond multiple=u32 5) -> ()  [unwired: 1 out]
                }
              }
              frame Enabled {
              }
            }
          }
          frame "Isquiotibiales" {
            n168 = Unbundle By Name(w438) -> ("Isquiotibiales"=w436:i32)
            n169 = To Unsigned Byte Integer(number=w436) -> (unsigned 8bit integer=w437:u8)
            n170 = Build Array(w437) -> (w442:u8[])
            n171 = Byte Array To String(unsigned byte array=w442) -> (string=w440:string)
            n172 = Concatenate Strings("2", w440) -> (w439:string)
            n173 = String Length(string=w439) -> (length=w445:i32)
            n174 = for {
              N: w445 -> [_]
              tunnel: w448 -> [w487]
              tunnel: w449 -> [w486]
              tunnel: w439 -> [w483]
              tunnel: [w480] -> w443
              tunnel: [w479] -> w444
              i -> [w481]
              n175 = String Subset(string=w483, offset (0)=w481, length (rest)=1 ("length (rest)")) -> (substring=w484:string)
              n176 = VISA Write(VISA resource name=w486, write buffer=w484, error in (no error)=w487) -> (VISA resource name out=w479:refnum<visa-resource-name>, error out=w480:errorcluster)  [unwired: 1 out]
              n177 = Wait Until Next ms Multiple(millisecond multiple=u32 5) -> ()  [unwired: 1 out]
            }
            n178 = disable-structure shown="Disabled" {
              disable-tunnel: [w461 w477] -> w447
              disable-tunnel: [w460 w478] -> w446
              disable-tunnel: w444 -> [w455 w478]
              disable-tunnel: w443 -> [w451 w477]
              frame Disabled {
                n179 = call "Timer2.vi"("error in (no error)"=w451, "Reset"=TRUE) -> ("error out"=w450:errorcluster)  [unwired: 7 in, 2 out]
                n180 = while {
                  tunnel: w455 -> [w467]
                  tunnel: [w467] -> w454
                  tunnel: [w465] -> w453
                  tunnel: w450 -> [w466]
                  stop <- w464 stop-if-true
                  n181 = call "Timer2.vi"("error in (no error)"=w466, "Time Target (s)"=0.25, "Pause"=TRUE) -> ("error out"=w465:errorcluster, "Time has Elapsed"=w464:bool)  [unwired: 6 in, 1 out]
                }
                n182 = property class="Instr"(reference=w454, error in=w453) -> (reference out=w458:refnum<visa-resource-name>, error out=w457:errorcluster, "Bytes at Port"=w456:u32)
                n183 = for {
                  N: w456 -> [_]
                  tunnel: w457 -> [w475]
                  tunnel: w458 -> [w474]
                  shift-right: [w469] -> _
                  shift-left: "" -> [w473]
                  tunnel: [w472] -> w461
                  tunnel: [w471] -> w460
                  n184 = VISA Read(VISA resource name=w474, byte count=u32 1, error in (no error)=w475) -> (VISA resource name out=w471:refnum<visa-resource-name>, read buffer=w468:string, error out=w472:errorcluster)  [unwired: 1 out]
                  n185 = Concatenate Strings(w473, w468) -> (w469:string)
                  n186 = Wait Until Next ms Multiple(millisecond multiple=u32 5) -> ()  [unwired: 1 out]
                }
              }
              frame Enabled {
              }
            }
          }
          frame "Gluteos" {
            n187 = Unbundle By Name(w490) -> ("Gluteos"=w488:i32)
            n188 = To Unsigned Byte Integer(number=w488) -> (unsigned 8bit integer=w489:u8)
            n189 = Build Array(w489) -> (w494:u8[])
            n190 = Byte Array To String(unsigned byte array=w494) -> (string=w492:string)
            n191 = Concatenate Strings("3", w492) -> (w491:string)
            n192 = String Length(string=w491) -> (length=w497:i32)
            n193 = for {
              N: w497 -> [_]
              tunnel: w500 -> [w539]
              tunnel: w501 -> [w538]
              tunnel: w491 -> [w535]
              tunnel: [w532] -> w495
              tunnel: [w531] -> w496
              i -> [w533]
              n194 = String Subset(string=w535, offset (0)=w533, length (rest)=1 ("length (rest)")) -> (substring=w536:string)
              n195 = VISA Write(VISA resource name=w538, write buffer=w536, error in (no error)=w539) -> (VISA resource name out=w531:refnum<visa-resource-name>, error out=w532:errorcluster)  [unwired: 1 out]
              n196 = Wait Until Next ms Multiple(millisecond multiple=u32 5) -> ()  [unwired: 1 out]
            }
            n197 = disable-structure shown="Disabled" {
              disable-tunnel: [w513 w529] -> w499
              disable-tunnel: [w512 w530] -> w498
              disable-tunnel: w496 -> [w507 w530]
              disable-tunnel: w495 -> [w503 w529]
              frame Disabled {
                n198 = call "Timer2.vi"("error in (no error)"=w503, "Reset"=TRUE) -> ("error out"=w502:errorcluster)  [unwired: 7 in, 2 out]
                n199 = while {
                  tunnel: w507 -> [w519]
                  tunnel: [w519] -> w506
                  tunnel: [w517] -> w505
                  tunnel: w502 -> [w518]
                  stop <- w516 stop-if-true
                  n200 = call "Timer2.vi"("error in (no error)"=w518, "Time Target (s)"=0.25, "Pause"=TRUE) -> ("error out"=w517:errorcluster, "Time has Elapsed"=w516:bool)  [unwired: 6 in, 1 out]
                }
                n201 = property class="Instr"(reference=w506, error in=w505) -> (reference out=w510:refnum<visa-resource-name>, error out=w509:errorcluster, "Bytes at Port"=w508:u32)
                n202 = for {
                  N: w508 -> [_]
                  tunnel: w509 -> [w527]
                  tunnel: w510 -> [w526]
                  shift-right: [w521] -> _
                  shift-left: "" -> [w525]
                  tunnel: [w524] -> w513
                  tunnel: [w523] -> w512
                  n203 = VISA Read(VISA resource name=w526, byte count=u32 1, error in (no error)=w527) -> (VISA resource name out=w523:refnum<visa-resource-name>, read buffer=w520:string, error out=w524:errorcluster)  [unwired: 1 out]
                  n204 = Concatenate Strings(w525, w520) -> (w521:string)
                  n205 = Wait Until Next ms Multiple(millisecond multiple=u32 5) -> ()  [unwired: 1 out]
                }
              }
              frame Enabled {
              }
            }
          }
          frame "Abdomen" {
            n206 = Unbundle By Name(w542) -> ("Abdomen"=w540:i32)
            n207 = To Unsigned Byte Integer(number=w540) -> (unsigned 8bit integer=w541:u8)
            n208 = Build Array(w541) -> (w546:u8[])
            n209 = Byte Array To String(unsigned byte array=w546) -> (string=w544:string)
            n210 = Concatenate Strings("4", w544) -> (w543:string)
            n211 = String Length(string=w543) -> (length=w549:i32)
            n212 = for {
              N: w549 -> [_]
              tunnel: w552 -> [w591]
              tunnel: w553 -> [w590]
              tunnel: w543 -> [w587]
              tunnel: [w584] -> w547
              tunnel: [w583] -> w548
              i -> [w585]
              n213 = String Subset(string=w587, offset (0)=w585, length (rest)=1 ("length (rest)")) -> (substring=w588:string)
              n214 = VISA Write(VISA resource name=w590, write buffer=w588, error in (no error)=w591) -> (VISA resource name out=w583:refnum<visa-resource-name>, error out=w584:errorcluster)  [unwired: 1 out]
              n215 = Wait Until Next ms Multiple(millisecond multiple=u32 5) -> ()  [unwired: 1 out]
            }
            n216 = disable-structure shown="Disabled" {
              disable-tunnel: [w565 w581] -> w551
              disable-tunnel: [w564 w582] -> w550
              disable-tunnel: w548 -> [w559 w582]
              disable-tunnel: w547 -> [w555 w581]
              frame Disabled {
                n217 = call "Timer2.vi"("error in (no error)"=w555, "Reset"=TRUE) -> ("error out"=w554:errorcluster)  [unwired: 7 in, 2 out]
                n218 = while {
                  tunnel: w559 -> [w571]
                  tunnel: [w571] -> w558
                  tunnel: [w569] -> w557
                  tunnel: w554 -> [w570]
                  stop <- w568 stop-if-true
                  n219 = call "Timer2.vi"("error in (no error)"=w570, "Time Target (s)"=0.25, "Pause"=TRUE) -> ("error out"=w569:errorcluster, "Time has Elapsed"=w568:bool)  [unwired: 6 in, 1 out]
                }
                n220 = property class="Instr"(reference=w558, error in=w557) -> (reference out=w562:refnum<visa-resource-name>, error out=w561:errorcluster, "Bytes at Port"=w560:u32)
                n221 = for {
                  N: w560 -> [_]
                  tunnel: w561 -> [w579]
                  tunnel: w562 -> [w578]
                  shift-right: [w573] -> _
                  shift-left: "" -> [w577]
                  tunnel: [w576] -> w565
                  tunnel: [w575] -> w564
                  n222 = VISA Read(VISA resource name=w578, byte count=u32 1, error in (no error)=w579) -> (VISA resource name out=w575:refnum<visa-resource-name>, read buffer=w572:string, error out=w576:errorcluster)  [unwired: 1 out]
                  n223 = Concatenate Strings(w577, w572) -> (w573:string)
                  n224 = Wait Until Next ms Multiple(millisecond multiple=u32 5) -> ()  [unwired: 1 out]
                }
              }
              frame Enabled {
              }
            }
          }
          frame "Lumbares" {
            n225 = Unbundle By Name(w594) -> ("Lumbares"=w592:i32)
            n226 = To Unsigned Byte Integer(number=w592) -> (unsigned 8bit integer=w593:u8)
            n227 = Build Array(w593) -> (w598:u8[])
            n228 = Byte Array To String(unsigned byte array=w598) -> (string=w596:string)
            n229 = Concatenate Strings("5", w596) -> (w595:string)
            n230 = String Length(string=w595) -> (length=w601:i32)
            n231 = for {
              N: w601 -> [_]
              tunnel: w604 -> [w643]
              tunnel: w605 -> [w642]
              tunnel: w595 -> [w639]
              tunnel: [w636] -> w599
              tunnel: [w635] -> w600
              i -> [w637]
              n232 = String Subset(string=w639, offset (0)=w637, length (rest)=1 ("length (rest)")) -> (substring=w640:string)
              n233 = VISA Write(VISA resource name=w642, write buffer=w640, error in (no error)=w643) -> (VISA resource name out=w635:refnum<visa-resource-name>, error out=w636:errorcluster)  [unwired: 1 out]
              n234 = Wait Until Next ms Multiple(millisecond multiple=u32 5) -> ()  [unwired: 1 out]
            }
            n235 = disable-structure shown="Disabled" {
              disable-tunnel: [w617 w633] -> w603
              disable-tunnel: [w616 w634] -> w602
              disable-tunnel: w600 -> [w611 w634]
              disable-tunnel: w599 -> [w607 w633]
              frame Disabled {
                n236 = call "Timer2.vi"("error in (no error)"=w607, "Reset"=TRUE) -> ("error out"=w606:errorcluster)  [unwired: 7 in, 2 out]
                n237 = while {
                  tunnel: w611 -> [w623]
                  tunnel: [w623] -> w610
                  tunnel: [w621] -> w609
                  tunnel: w606 -> [w622]
                  stop <- w620 stop-if-true
                  n238 = call "Timer2.vi"("error in (no error)"=w622, "Time Target (s)"=0.25, "Pause"=TRUE) -> ("error out"=w621:errorcluster, "Time has Elapsed"=w620:bool)  [unwired: 6 in, 1 out]
                }
                n239 = property class="Instr"(reference=w610, error in=w609) -> (reference out=w614:refnum<visa-resource-name>, error out=w613:errorcluster, "Bytes at Port"=w612:u32)
                n240 = for {
                  N: w612 -> [_]
                  tunnel: w613 -> [w631]
                  tunnel: w614 -> [w630]
                  shift-right: [w625] -> _
                  shift-left: "" -> [w629]
                  tunnel: [w628] -> w617
                  tunnel: [w627] -> w616
                  n241 = VISA Read(VISA resource name=w630, byte count=u32 1, error in (no error)=w631) -> (VISA resource name out=w627:refnum<visa-resource-name>, read buffer=w624:string, error out=w628:errorcluster)  [unwired: 1 out]
                  n242 = Concatenate Strings(w629, w624) -> (w625:string)
                  n243 = Wait Until Next ms Multiple(millisecond multiple=u32 5) -> ()  [unwired: 1 out]
                }
              }
              frame Enabled {
              }
            }
          }
          frame "Dorsales" {
            n244 = Unbundle By Name(w646) -> ("Dorsales"=w644:i32)
            n245 = To Unsigned Byte Integer(number=w644) -> (unsigned 8bit integer=w645:u8)
            n246 = Build Array(w645) -> (w650:u8[])
            n247 = Byte Array To String(unsigned byte array=w650) -> (string=w648:string)
            n248 = Concatenate Strings("6", w648) -> (w647:string)
            n249 = String Length(string=w647) -> (length=w653:i32)
            n250 = for {
              N: w653 -> [_]
              tunnel: w656 -> [w695]
              tunnel: w657 -> [w694]
              tunnel: w647 -> [w691]
              tunnel: [w688] -> w651
              tunnel: [w687] -> w652
              i -> [w689]
              n251 = String Subset(string=w691, offset (0)=w689, length (rest)=1 ("length (rest)")) -> (substring=w692:string)
              n252 = VISA Write(VISA resource name=w694, write buffer=w692, error in (no error)=w695) -> (VISA resource name out=w687:refnum<visa-resource-name>, error out=w688:errorcluster)  [unwired: 1 out]
              n253 = Wait Until Next ms Multiple(millisecond multiple=u32 5) -> ()  [unwired: 1 out]
            }
            n254 = disable-structure shown="Disabled" {
              disable-tunnel: [w669 w685] -> w655
              disable-tunnel: [w668 w686] -> w654
              disable-tunnel: w652 -> [w663 w686]
              disable-tunnel: w651 -> [w659 w685]
              frame Disabled {
                n255 = call "Timer2.vi"("error in (no error)"=w659, "Reset"=TRUE) -> ("error out"=w658:errorcluster)  [unwired: 7 in, 2 out]
                n256 = while {
                  tunnel: w663 -> [w675]
                  tunnel: [w675] -> w662
                  tunnel: [w673] -> w661
                  tunnel: w658 -> [w674]
                  stop <- w672 stop-if-true
                  n257 = call "Timer2.vi"("error in (no error)"=w674, "Time Target (s)"=0.25, "Pause"=TRUE) -> ("error out"=w673:errorcluster, "Time has Elapsed"=w672:bool)  [unwired: 6 in, 1 out]
                }
                n258 = property class="Instr"(reference=w662, error in=w661) -> (reference out=w666:refnum<visa-resource-name>, error out=w665:errorcluster, "Bytes at Port"=w664:u32)
                n259 = for {
                  N: w664 -> [_]
                  tunnel: w665 -> [w683]
                  tunnel: w666 -> [w682]
                  shift-right: [w677] -> _
                  shift-left: "" -> [w681]
                  tunnel: [w680] -> w669
                  tunnel: [w679] -> w668
                  n260 = VISA Read(VISA resource name=w682, byte count=u32 1, error in (no error)=w683) -> (VISA resource name out=w679:refnum<visa-resource-name>, read buffer=w676:string, error out=w680:errorcluster)  [unwired: 1 out]
                  n261 = Concatenate Strings(w681, w676) -> (w677:string)
                  n262 = Wait Until Next ms Multiple(millisecond multiple=u32 5) -> ()  [unwired: 1 out]
                }
              }
              frame Enabled {
              }
            }
          }
          frame "Trapecio" {
            n263 = Unbundle By Name(w698) -> ("Trapecio"=w696:i32)
            n264 = To Unsigned Byte Integer(number=w696) -> (unsigned 8bit integer=w697:u8)
            n265 = Build Array(w697) -> (w702:u8[])
            n266 = Byte Array To String(unsigned byte array=w702) -> (string=w700:string)
            n267 = Concatenate Strings("7", w700) -> (w699:string)
            n268 = String Length(string=w699) -> (length=w705:i32)
            n269 = for {
              N: w705 -> [_]
              tunnel: w708 -> [w747]
              tunnel: w709 -> [w746]
              tunnel: w699 -> [w743]
              tunnel: [w740] -> w703
              tunnel: [w739] -> w704
              i -> [w741]
              n270 = String Subset(string=w743, offset (0)=w741, length (rest)=1 ("length (rest)")) -> (substring=w744:string)
              n271 = VISA Write(VISA resource name=w746, write buffer=w744, error in (no error)=w747) -> (VISA resource name out=w739:refnum<visa-resource-name>, error out=w740:errorcluster)  [unwired: 1 out]
              n272 = Wait Until Next ms Multiple(millisecond multiple=u32 5) -> ()  [unwired: 1 out]
            }
            n273 = disable-structure shown="Disabled" {
              disable-tunnel: [w721 w737] -> w707
              disable-tunnel: [w720 w738] -> w706
              disable-tunnel: w704 -> [w715 w738]
              disable-tunnel: w703 -> [w711 w737]
              frame Disabled {
                n274 = call "Timer2.vi"("error in (no error)"=w711, "Reset"=TRUE) -> ("error out"=w710:errorcluster)  [unwired: 7 in, 2 out]
                n275 = while {
                  tunnel: w715 -> [w727]
                  tunnel: [w727] -> w714
                  tunnel: [w725] -> w713
                  tunnel: w710 -> [w726]
                  stop <- w724 stop-if-true
                  n276 = call "Timer2.vi"("error in (no error)"=w726, "Time Target (s)"=0.25, "Pause"=TRUE) -> ("error out"=w725:errorcluster, "Time has Elapsed"=w724:bool)  [unwired: 6 in, 1 out]
                }
                n277 = property class="Instr"(reference=w714, error in=w713) -> (reference out=w718:refnum<visa-resource-name>, error out=w717:errorcluster, "Bytes at Port"=w716:u32)
                n278 = for {
                  N: w716 -> [_]
                  tunnel: w717 -> [w735]
                  tunnel: w718 -> [w734]
                  shift-right: [w729] -> _
                  shift-left: "" -> [w733]
                  tunnel: [w732] -> w721
                  tunnel: [w731] -> w720
                  n279 = VISA Read(VISA resource name=w734, byte count=u32 1, error in (no error)=w735) -> (VISA resource name out=w731:refnum<visa-resource-name>, read buffer=w728:string, error out=w732:errorcluster)  [unwired: 1 out]
                  n280 = Concatenate Strings(w733, w728) -> (w729:string)
                  n281 = Wait Until Next ms Multiple(millisecond multiple=u32 5) -> ()  [unwired: 1 out]
                }
              }
              frame Enabled {
              }
            }
          }
          frame "Pectorales" {
            n282 = Unbundle By Name(w750) -> ("Pectorales"=w748:i32)
            n283 = To Unsigned Byte Integer(number=w748) -> (unsigned 8bit integer=w749:u8)
            n284 = Build Array(w749) -> (w754:u8[])
            n285 = Byte Array To String(unsigned byte array=w754) -> (string=w752:string)
            n286 = Concatenate Strings("8", w752) -> (w751:string)
            n287 = String Length(string=w751) -> (length=w757:i32)
            n288 = for {
              N: w757 -> [_]
              tunnel: w760 -> [w799]
              tunnel: w761 -> [w798]
              tunnel: w751 -> [w795]
              tunnel: [w792] -> w755
              tunnel: [w791] -> w756
              i -> [w793]
              n289 = String Subset(string=w795, offset (0)=w793, length (rest)=1 ("length (rest)")) -> (substring=w796:string)
              n290 = VISA Write(VISA resource name=w798, write buffer=w796, error in (no error)=w799) -> (VISA resource name out=w791:refnum<visa-resource-name>, error out=w792:errorcluster)  [unwired: 1 out]
              n291 = Wait Until Next ms Multiple(millisecond multiple=u32 5) -> ()  [unwired: 1 out]
            }
            n292 = disable-structure shown="Disabled" {
              disable-tunnel: [w773 w789] -> w759
              disable-tunnel: [w772 w790] -> w758
              disable-tunnel: w756 -> [w767 w790]
              disable-tunnel: w755 -> [w763 w789]
              frame Disabled {
                n293 = call "Timer2.vi"("error in (no error)"=w763, "Reset"=TRUE) -> ("error out"=w762:errorcluster)  [unwired: 7 in, 2 out]
                n294 = while {
                  tunnel: w767 -> [w779]
                  tunnel: [w779] -> w766
                  tunnel: [w777] -> w765
                  tunnel: w762 -> [w778]
                  stop <- w776 stop-if-true
                  n295 = call "Timer2.vi"("error in (no error)"=w778, "Time Target (s)"=0.25, "Pause"=TRUE) -> ("error out"=w777:errorcluster, "Time has Elapsed"=w776:bool)  [unwired: 6 in, 1 out]
                }
                n296 = property class="Instr"(reference=w766, error in=w765) -> (reference out=w770:refnum<visa-resource-name>, error out=w769:errorcluster, "Bytes at Port"=w768:u32)
                n297 = for {
                  N: w768 -> [_]
                  tunnel: w769 -> [w787]
                  tunnel: w770 -> [w786]
                  shift-right: [w781] -> _
                  shift-left: "" -> [w785]
                  tunnel: [w784] -> w773
                  tunnel: [w783] -> w772
                  n298 = VISA Read(VISA resource name=w786, byte count=u32 1, error in (no error)=w787) -> (VISA resource name out=w783:refnum<visa-resource-name>, read buffer=w780:string, error out=w784:errorcluster)  [unwired: 1 out]
                  n299 = Concatenate Strings(w785, w780) -> (w781:string)
                  n300 = Wait Until Next ms Multiple(millisecond multiple=u32 5) -> ()  [unwired: 1 out]
                }
              }
              frame Enabled {
              }
            }
          }
          frame "Biceps" {
            n301 = Unbundle By Name(w802) -> ("Biceps"=w800:i32)
            n302 = To Unsigned Byte Integer(number=w800) -> (unsigned 8bit integer=w801:u8)
            n303 = Build Array(w801) -> (w806:u8[])
            n304 = Byte Array To String(unsigned byte array=w806) -> (string=w804:string)
            n305 = Concatenate Strings("9", w804) -> (w803:string)
            n306 = String Length(string=w803) -> (length=w809:i32)
            n307 = for {
              N: w809 -> [_]
              tunnel: w812 -> [w851]
              tunnel: w813 -> [w850]
              tunnel: w803 -> [w847]
              tunnel: [w844] -> w807
              tunnel: [w843] -> w808
              i -> [w845]
              n308 = String Subset(string=w847, offset (0)=w845, length (rest)=1 ("length (rest)")) -> (substring=w848:string)
              n309 = VISA Write(VISA resource name=w850, write buffer=w848, error in (no error)=w851) -> (VISA resource name out=w843:refnum<visa-resource-name>, error out=w844:errorcluster)  [unwired: 1 out]
              n310 = Wait Until Next ms Multiple(millisecond multiple=u32 5) -> ()  [unwired: 1 out]
            }
            n311 = disable-structure shown="Disabled" {
              disable-tunnel: [w825 w841] -> w811
              disable-tunnel: [w824 w842] -> w810
              disable-tunnel: w808 -> [w819 w842]
              disable-tunnel: w807 -> [w815 w841]
              frame Disabled {
                n312 = call "Timer2.vi"("error in (no error)"=w815, "Reset"=TRUE) -> ("error out"=w814:errorcluster)  [unwired: 7 in, 2 out]
                n313 = while {
                  tunnel: w819 -> [w831]
                  tunnel: [w831] -> w818
                  tunnel: [w829] -> w817
                  tunnel: w814 -> [w830]
                  stop <- w828 stop-if-true
                  n314 = call "Timer2.vi"("error in (no error)"=w830, "Time Target (s)"=0.25, "Pause"=TRUE) -> ("error out"=w829:errorcluster, "Time has Elapsed"=w828:bool)  [unwired: 6 in, 1 out]
                }
                n315 = property class="Instr"(reference=w818, error in=w817) -> (reference out=w822:refnum<visa-resource-name>, error out=w821:errorcluster, "Bytes at Port"=w820:u32)
                n316 = for {
                  N: w820 -> [_]
                  tunnel: w821 -> [w839]
                  tunnel: w822 -> [w838]
                  shift-right: [w833] -> _
                  shift-left: "" -> [w837]
                  tunnel: [w836] -> w825
                  tunnel: [w835] -> w824
                  n317 = VISA Read(VISA resource name=w838, byte count=u32 1, error in (no error)=w839) -> (VISA resource name out=w835:refnum<visa-resource-name>, read buffer=w832:string, error out=w836:errorcluster)  [unwired: 1 out]
                  n318 = Concatenate Strings(w837, w832) -> (w833:string)
                  n319 = Wait Until Next ms Multiple(millisecond multiple=u32 5) -> ()  [unwired: 1 out]
                }
              }
              frame Enabled {
              }
            }
          }
          frame "Opcional" {
            n320 = Unbundle By Name(w854) -> ("Opcional"=w852:i32)
            n321 = To Unsigned Byte Integer(number=w852) -> (unsigned 8bit integer=w853:u8)
            n322 = Build Array(w853) -> (w858:u8[])
            n323 = Byte Array To String(unsigned byte array=w858) -> (string=w856:string)
            n324 = Concatenate Strings("10", w856) -> (w855:string)
            n325 = String Length(string=w855) -> (length=w861:i32)
            n326 = for {
              N: w861 -> [_]
              tunnel: w864 -> [w903]
              tunnel: w865 -> [w902]
              tunnel: w855 -> [w899]
              tunnel: [w896] -> w859
              tunnel: [w895] -> w860
              i -> [w897]
              n327 = String Subset(string=w899, offset (0)=w897, length (rest)=1 ("length (rest)")) -> (substring=w900:string)
              n328 = VISA Write(VISA resource name=w902, write buffer=w900, error in (no error)=w903) -> (VISA resource name out=w895:refnum<visa-resource-name>, error out=w896:errorcluster)  [unwired: 1 out]
              n329 = Wait Until Next ms Multiple(millisecond multiple=u32 5) -> ()  [unwired: 1 out]
            }
            n330 = disable-structure shown="Disabled" {
              disable-tunnel: [w877 w893] -> w863
              disable-tunnel: [w876 w894] -> w862
              disable-tunnel: w860 -> [w871 w894]
              disable-tunnel: w859 -> [w867 w893]
              frame Disabled {
                n331 = call "Timer2.vi"("error in (no error)"=w867, "Reset"=TRUE) -> ("error out"=w866:errorcluster)  [unwired: 7 in, 2 out]
                n332 = while {
                  tunnel: w871 -> [w883]
                  tunnel: [w883] -> w870
                  tunnel: [w881] -> w869
                  tunnel: w866 -> [w882]
                  stop <- w880 stop-if-true
                  n333 = call "Timer2.vi"("error in (no error)"=w882, "Time Target (s)"=0.25, "Pause"=TRUE) -> ("error out"=w881:errorcluster, "Time has Elapsed"=w880:bool)  [unwired: 6 in, 1 out]
                }
                n334 = property class="Instr"(reference=w870, error in=w869) -> (reference out=w874:refnum<visa-resource-name>, error out=w873:errorcluster, "Bytes at Port"=w872:u32)
                n335 = for {
                  N: w872 -> [_]
                  tunnel: w873 -> [w891]
                  tunnel: w874 -> [w890]
                  shift-right: [w885] -> _
                  shift-left: "" -> [w889]
                  tunnel: [w888] -> w877
                  tunnel: [w887] -> w876
                  n336 = VISA Read(VISA resource name=w890, byte count=u32 1, error in (no error)=w891) -> (VISA resource name out=w887:refnum<visa-resource-name>, read buffer=w884:string, error out=w888:errorcluster)  [unwired: 1 out]
                  n337 = Concatenate Strings(w889, w884) -> (w885:string)
                  n338 = Wait Until Next ms Multiple(millisecond multiple=u32 5) -> ()  [unwired: 1 out]
                }
              }
              frame Enabled {
              }
            }
          }
        }
      }
      frame Error {
        # "Return true in any case that should stop the loop."
      }
    }
  }
  n339 = while {
    tunnel: w15 -> [_]
    tunnel: w8 -> [w911]
    shift-right: [w909] -> _
    shift-left: w10 -> [w910]
    shift-right: [w907] -> w2
    shift-left: w3 -> [w908]
    stop <- w913 stop-if-true
    n340 = event shown="[0] Timeout" {
      selector: _ -> [_ _ _ _ _ _ _ _ _ _ _ _ _ _ _ _ _ _ _ _]
      dyn-events: _ -> [_ _ _ _ _ _ _ _ _ _ _ _ _ _ _ _ _ _ _ _]
      timeout: 300 -> [_ _ _ _ _ _ _ _ _ _ _ _ _ _ _ _ _ _ _ _]
      tunnel: [w919 FALSE FALSE FALSE FALSE FALSE FALSE FALSE FALSE FALSE FALSE _ _ _ TRUE ("Stop") FALSE ("Stop") FALSE ("Stop") FALSE ("Stop") FALSE ("Stop") FALSE ("Stop")] -> w913
      tunnel: w911 -> [w917 _ _ _ _ _ _ _ _ _ _ w1288 w1438 w1553 _ _ _ w1691 w1743 w1749]
      tunnel: w910 -> [w915 w1049 w1074 w1100 w1125 w1150 w1175 w1200 w1225 w1250 w1275 w1291 w1440 w1557 w1630 w1633 w1662 w1671 w1744 w1753]
      tunnel: [w914 w1050 w1075 w1099 w1124 w1149 w1174 w1199 w1224 w1249 w1274 w1292 w1441 w1558 w1628 w1632 w1662 w1676 w1695 w1752] -> w909
      tunnel: w908 -> [w916 _ _ _ _ _ _ _ _ _ _ w1289 w1437 w1554 _ _ _ w1690 w1742 w1748]
      tunnel: [_ _ _ _ _ _ _ _ _ _ _ _ _ _ _ _ _ w1678 _ w1747] -> w907
      event Timeout {
        n341 = event-data() -> ()  [unwired: 1 in, 3 out]
        n342 = Unbundle By Name(w915) -> ("Label"=w935:string, "Cuadriceps"=w934:i32, "Isquiotibiales"=w933:i32, "Gluteos"=w932:i32, "Abdomen"=w931:i32, "Lumbares"=w930:i32, "Dorsales"=w929:i32, "Trapecio"=w928:i32, "Pectorales"=w927:i32, "Biceps"=w926:i32, "Opcional"=w925:i32, "Master"=w921:i32, "Slider"=w920:i32)
        n343 = Unbundle By Name(w915) -> ("Impulso"=w923:i32, "Tiempo"=w922:i32)
        n344 = Format Date/Time String() -> (date/time string=→"date/time string":string)  [unwired: 3 in]
        n345 = local read "Start?"() -> (w936:bool)
        n346 = case shown="\"Cuadriceps\"" w935 {
          selector: w935 -> [w985 w990 w995 w1000 w1005 w1010 w1015 w1020 w1025 w1030 w1035 w1037]
          tunnel: [w985 w990 w995 w1000 w1005 w1010 w1015 w1020 w1025 w1030 w1035 w1037] -> _
          tunnel: [w981 w986 w991 w996 w1001 w1006 w1011 w1016 w1021 w1026 w1031 w1036] -> w924
          tunnel: w934 -> [w981 _ _ _ _ _ _ _ _ _ _ _]
          tunnel: w933 -> [_ w986 _ _ _ _ _ _ _ _ _ _]
          tunnel: w932 -> [_ _ w991 _ _ _ _ _ _ _ _ _]
          tunnel: w931 -> [_ _ _ w996 _ _ _ _ _ _ _ _]
          tunnel: w930 -> [_ _ _ _ w1001 _ _ _ _ _ _ _]
          tunnel: w929 -> [_ _ _ _ _ w1006 _ _ _ _ _ _]
          tunnel: w928 -> [_ _ _ _ _ _ w1011 _ _ _ _ _]
          tunnel: w927 -> [_ _ _ _ _ _ _ w1016 _ _ _ _]
          tunnel: w926 -> [_ _ _ _ _ _ _ _ w1021 _ _ _]
          tunnel: w925 -> [_ _ _ _ _ _ _ _ _ w1026 _ _]
          tunnel: w921 -> [_ _ _ _ _ _ _ _ _ _ w1031 _]
          tunnel: w920 -> [_ _ _ _ _ _ _ _ _ _ _ w1036]
          frame "Cuadriceps" {
            n347 = Number To Decimal String(number=w981) -> (decimal integer string=w984:string)  [unwired: 1 in]
            n348 = Concatenate Strings(w984, "%" ("string")) -> (→"Cuadríceps %":string)
          }
          frame "Isquiotibiales" {
            n349 = Number To Decimal String(number=w986) -> (decimal integer string=w989:string)  [unwired: 1 in]
            n350 = Concatenate Strings(w989, "%" ("string")) -> (→"Isquiotibiales %":string)
          }
          frame "Gluteos" {
            n351 = Number To Decimal String(number=w991) -> (decimal integer string=w994:string)  [unwired: 1 in]
            n352 = Concatenate Strings(w994, "%" ("string")) -> (→"Gluteos %":string)
          }
          frame "Abdomen" {
            n353 = Number To Decimal String(number=w996) -> (decimal integer string=w999:string)  [unwired: 1 in]
            n354 = Concatenate Strings(w999, "%" ("string")) -> (→"Abdomen %":string)
          }
          frame "Lumbares" {
            n355 = Number To Decimal String(number=w1001) -> (decimal integer string=w1004:string)  [unwired: 1 in]
            n356 = Concatenate Strings(w1004, "%" ("string")) -> (→"Lumbares %":string)
          }
          frame "Dorsales" {
            n357 = Number To Decimal String(number=w1006) -> (decimal integer string=w1009:string)  [unwired: 1 in]
            n358 = Concatenate Strings(w1009, "%" ("string")) -> (→"Dorsales %":string)
          }
          frame "Trapecio" {
            n359 = Number To Decimal String(number=w1011) -> (decimal integer string=w1014:string)  [unwired: 1 in]
            n360 = Concatenate Strings(w1014, "%" ("string")) -> (→"Trapecio %":string)
          }
          frame "Pectorales" {
            n361 = Number To Decimal String(number=w1016) -> (decimal integer string=w1019:string)  [unwired: 1 in]
            n362 = Concatenate Strings(w1019, "%" ("string")) -> (→"Pectorales %":string)
          }
          frame "Biceps" {
            n363 = Number To Decimal String(number=w1021) -> (decimal integer string=w1024:string)  [unwired: 1 in]
            n364 = Concatenate Strings(w1024, "%" ("string")) -> (→"Biceps %":string)
          }
          frame "Opcional" {
            n365 = Number To Decimal String(number=w1026) -> (decimal integer string=w1029:string)  [unwired: 1 in]
            n366 = Concatenate Strings(w1029, "%" ("string")) -> (→"Opcional %":string)
          }
          frame "Master" {
            n367 = Number To Decimal String(number=w1031) -> (decimal integer string=w1034:string)  [unwired: 1 in]
            n368 = Concatenate Strings(w1034, "%" ("string")) -> (→"Master Ind":string)
          }
          frame "Inicio", Default {
          }
        }
        "Horizontal Graduated Bar" <- w924
        n369 = case shown="True" w936 {
          tunnel: w922 -> [_ w953]
          tunnel: w923 -> [_ w952]
          tunnel: [_ w942] -> w919
          tunnel: w915 -> [_ w951]
          tunnel: w917 -> [_ w947]
          tunnel: w916 -> [_ w946]
          tunnel: w915 -> [w937 w945]
          tunnel: [w937 w944] -> w914
          frame False {
            n370 = property on="Start" class="Bool (strict)"("BoolText.Text"="Start / Inicio" ("Boolean Text.Text")) -> ()  [unwired: 2 in, 2 out]
            n371 = flat-sequence {
              tunnel: [w939] -> _
              frame #0 {
                w939 = FALSE ("Visible")
                n372 = property on="Tiempo Restante" class="Str"("Visible"=w939) -> (error out=w940:errorcluster)  [unwired: 2 in, 1 out]
                n373 = property on="Tiempo Transcurrido" class="Str"(error in=w940, "Visible"=w939) -> ()  [unwired: 1 in, 2 out]
              }
            }
          }
          frame True {
            n374 = Unbundle By Name(w951) -> ("Label"=w948:string, "Impulso"=w950:i32, "Ruptura"=w949:i32)
            n375 = Number To Decimal String(number=w952) -> (decimal integer string=→"Hola":string)  [unwired: 1 in]
            n376 = Multiply(x=w953, y=60) -> (x*y=w943:i32)
            n377 = property on="Start" class="Bool (strict)"("BoolText.Text"="Stop / Parar" ("Boolean Text.Text")) -> ()  [unwired: 2 in, 2 out]
            n378 = call "Elapsed Time"("Time Target (s)"=w943) -> ("Elapsed Time (s)"=w941:dbl, "Time has Elapsed"=w942:bool)  [unwired: 11 in, 6 out]
            n379 = Subtract(x=w943, y=w941) -> (x-y=w960:dbl)
            n380 = To Time Stamp(1:w960) -> (0:w957:timestamp)
            n381 = To Time Stamp(1:w941) -> (0:w961:timestamp)
            n382 = Format Date/Time String(time format string (%c)="%M : %S", seconds (now)=w957) -> (date/time string=→"Tiempo Restante":string)  [unwired: 1 in]
            n383 = case shown="\"Encender\"" w948 {
              tunnel: w950 -> [w971 w978 _]
              tunnel: w949 -> [w970 w977 _]
              tunnel: w947 -> [w969 w976 _]
              tunnel: w946 -> [w968 w975 _]
              tunnel: w945 -> [w967 w974 w980]
              tunnel: [w966 w973 w980] -> w944
              frame "Start" {
                n384 = Bundle By Name(cluster=w967, "Label"="Encender", "Impulso"=w971, "Ruptura"=w970) -> (w966:T2)
                n385 = Enqueue Element(queue=w969, element=w966, error in (no error)=w968) -> ()  [unwired: 1 in, 3 out]
              }
              frame "Encender" {
                n386 = Bundle By Name(cluster=w974, "Label"="Encender", "Impulso"=w978, "Ruptura"=w977) -> (w973:T2)
                n387 = Enqueue Element(queue=w976, element=w973, error in (no error)=w975) -> ()  [unwired: 1 in, 3 out]
              }
              frame "Inicio", Default {
              }
            }
            n388 = Format Date/Time String(time format string (%c)="%M : %S", seconds (now)=w961) -> (date/time string=→"Tiempo Transcurrido":string)  [unwired: 1 in]
            n389 = flat-sequence {
              tunnel: [w964] -> _
              frame #0 {
                w964 = TRUE ("Visible")
                n390 = property on="Tiempo Restante" class="Str"("Visible"=w964) -> (error out=w965:errorcluster)  [unwired: 2 in, 1 out]
                n391 = property on="Tiempo Transcurrido" class="Str"(error in=w965, "Visible"=w964) -> ()  [unwired: 1 in, 2 out]
              }
            }
          }
        }
        n392 = local write "Slider"(w924) -> ()
      }
      event "Cuadriceps Bool": Value Change {
        n393 = event-data() -> ()  [unwired: 1 in, 6 out]
        n394 = Bundle By Name(cluster=cluster{"Color Box":u32, "Color Box 2":u32} {"Color Box"=12369084, "Color Box 2"=12369084}, "Color Box"=u32 16711680 ("Color Box 2")) -> (w1059:cluster{"Color Box":u32, "Color Box 2":u32})
        n395 = Bundle By Name(cluster=cluster{"Color Box":u32, "Color Box 2":u32} {"Color Box"=12369084, "Color Box 2"=12369084}, "Color Box"=u32 12369084 ("Color Box 2")) -> (w1054:cluster{"Color Box":u32, "Color Box 2":u32})
        n396 = Bundle By Name(cluster=w1049, "Label"="Cuadriceps" ("Message")) -> (w1050:T2)
        n397 = property on="Master" class="Bool (strict)"() -> (error out=w1039:errorcluster, "Colors [4]"=w1042:cluster{u32, u32}[])  [unwired: 2 in, 1 out]
        n398 = Insert Into Array(array=cluster{u32, u32}[] [] ("Colors [4]"), new element=w1059) -> (w1058:cluster{u32, u32}[])  [unwired: 1 in]
        n399 = Insert Into Array(array=cluster{u32, u32}[] [] ("Colors [4]"), new element=w1054) -> (w1052:cluster{u32, u32}[])  [unwired: 1 in]
        n400 = Index Array(array=w1042) -> (element=w1048:cluster{u32, u32})  [unwired: 1 in]
        n401 = property on="Cuadriceps Bool" class="Bool"("Colors [4]"=w1058) -> ()  [unwired: 2 in, 2 out]
        n402 = Unbundle(w1048) -> (w1044:u32)  [unwired: 1 out]
        n403 = property on="Abdomen Bool" class="Bool"("Colors [4]"=w1052) -> ()  [unwired: 2 in, 2 out]
        n404 = property on="Lumbares Bool" class="Bool"("Colors [4]"=w1052) -> ()  [unwired: 2 in, 2 out]
        n405 = property on="Gluteos Bool" class="Bool"("Colors [4]"=w1052) -> ()  [unwired: 2 in, 2 out]
        n406 = property on="Isquiotibiales Bool" class="Bool"("Colors [4]"=w1052) -> ()  [unwired: 2 in, 2 out]
        n407 = Bundle(w1044, "Boolean Text.Text Colors:Text Color"=u32 40709) -> (w1047:T3)  [unwired: 1 in]
        n408 = property on="Pectorales Bool" class="Bool"("Colors [4]"=w1052) -> ()  [unwired: 2 in, 2 out]
        n409 = property on="Dorsales Bool" class="Bool"("Colors [4]"=w1052) -> ()  [unwired: 2 in, 2 out]
        n410 = property on="Trapecio Bool" class="Bool"("Colors [4]"=w1052) -> ()  [unwired: 2 in, 2 out]
        n411 = property on="Opcional Bool" class="Bool"("Colors [4]"=w1052) -> ()  [unwired: 2 in, 2 out]
        n412 = property on="Biceps Bool" class="Bool"("Colors [4]"=w1052) -> ()  [unwired: 2 in, 2 out]
        n413 = Replace Array Subset(array=w1042, new element=w1047, index=0) -> (w1041:cluster{u32, u32}[])
        n414 = property on="Master" class="Bool (strict)"(error in=w1039, "Colors [4]"=w1041) -> (error out=w1040:errorcluster)  [unwired: 1 in, 1 out]
        n415 = local write "Master"(FALSE ("Master")) -> ()
        n416 = property on="Master" class="Bool (strict)"(error in=w1040, "BoolText.TextColor"=u32 16448250 ("Boolean Text.Text Colors:Text Color")) -> ()  [unwired: 1 in, 2 out]
      }
      event "Isquiotibiales Bool": Value Change {
        n417 = event-data() -> ()  [unwired: 1 in, 6 out]
        n418 = Bundle By Name(cluster=cluster{"Color Box":u32, "Color Box 2":u32} {"Color Box"=12369084, "Color Box 2"=12369084}, "Color Box"=u32 16711680 ("Color Box 2")) -> (w1084:cluster{"Color Box":u32, "Color Box 2":u32})
        n419 = Bundle By Name(cluster=cluster{"Color Box":u32, "Color Box 2":u32} {"Color Box"=12369084, "Color Box 2"=12369084}, "Color Box"=u32 12369084 ("Color Box 2")) -> (w1080:cluster{"Color Box":u32, "Color Box 2":u32})
        n420 = Bundle By Name(cluster=w1074, "Label"="Isquiotibiales" ("Message")) -> (w1075:T2)
        n421 = property on="Master" class="Bool (strict)"() -> (error out=w1064:errorcluster, "Colors [4]"=w1067:cluster{u32, u32}[])  [unwired: 2 in, 1 out]
        n422 = Insert Into Array(array=cluster{u32, u32}[] [] ("Colors [4]"), new element=w1084) -> (w1078:cluster{u32, u32}[])  [unwired: 1 in]
        n423 = Insert Into Array(array=cluster{u32, u32}[] [] ("Colors [4]"), new element=w1080) -> (w1077:cluster{u32, u32}[])  [unwired: 1 in]
        n424 = local write "Master"(FALSE ("Master")) -> ()
        n425 = Index Array(array=w1067) -> (element=w1073:cluster{u32, u32})  [unwired: 1 in]
        n426 = property on="Isquiotibiales Bool" class="Bool"("Colors [4]"=w1078) -> ()  [unwired: 2 in, 2 out]
        n427 = property on="Abdomen Bool" class="Bool"("Colors [4]"=w1077) -> ()  [unwired: 2 in, 2 out]
        n428 = property on="Lumbares Bool" class="Bool"("Colors [4]"=w1077) -> ()  [unwired: 2 in, 2 out]
        n429 = property on="Gluteos Bool" class="Bool"("Colors [4]"=w1077) -> ()  [unwired: 2 in, 2 out]
        n430 = property on="Cuadriceps Bool" class="Bool"("Colors [4]"=w1077) -> ()  [unwired: 2 in, 2 out]
        n431 = Unbundle(w1073) -> (w1069:u32)  [unwired: 1 out]
        n432 = Bundle(w1069, "Boolean Text.Text Colors:Text Color"=u32 40709) -> (w1072:T3)  [unwired: 1 in]
        n433 = property on="Pectorales Bool" class="Bool"("Colors [4]"=w1077) -> ()  [unwired: 2 in, 2 out]
        n434 = property on="Dorsales Bool" class="Bool"("Colors [4]"=w1077) -> ()  [unwired: 2 in, 2 out]
        n435 = property on="Trapecio Bool" class="Bool"("Colors [4]"=w1077) -> ()  [unwired: 2 in, 2 out]
        n436 = property on="Opcional Bool" class="Bool"("Colors [4]"=w1077) -> ()  [unwired: 2 in, 2 out]
        n437 = property on="Biceps Bool" class="Bool"("Colors [4]"=w1077) -> ()  [unwired: 2 in, 2 out]
        n438 = Replace Array Subset(array=w1067, new element=w1072, index=0) -> (w1066:cluster{u32, u32}[])
        n439 = property on="Master" class="Bool (strict)"(error in=w1064, "Colors [4]"=w1066) -> (error out=w1065:errorcluster)  [unwired: 1 in, 1 out]
        n440 = property on="Master" class="Bool (strict)"(error in=w1065, "BoolText.TextColor"=u32 16448250 ("Boolean Text.Text Colors:Text Color")) -> ()  [unwired: 1 in, 2 out]
      }
      event "Gluteos Bool": Value Change {
        n441 = event-data() -> ()  [unwired: 1 in, 6 out]
        n442 = Bundle By Name(cluster=cluster{"Color Box":u32, "Color Box 2":u32} {"Color Box"=12369084, "Color Box 2"=12369084}, "Color Box"=u32 16711680 ("Color Box 2")) -> (w1109:cluster{"Color Box":u32, "Color Box 2":u32})
        n443 = Bundle By Name(cluster=cluster{"Color Box":u32, "Color Box 2":u32} {"Color Box"=12369084, "Color Box 2"=12369084}, "Color Box"=u32 12369084 ("Color Box 2")) -> (w1105:cluster{"Color Box":u32, "Color Box 2":u32})
        n444 = Bundle By Name(cluster=w1100, "Label"="Gluteos" ("Message")) -> (w1099:T2)
        n445 = property on="Master" class="Bool (strict)"() -> (error out=w1089:errorcluster, "Colors [4]"=w1092:cluster{u32, u32}[])  [unwired: 2 in, 1 out]
        n446 = Insert Into Array(array=cluster{u32, u32}[] [] ("Colors [4]"), new element=w1109) -> (w1103:cluster{u32, u32}[])  [unwired: 1 in]
        n447 = Insert Into Array(array=cluster{u32, u32}[] [] ("Colors [4]"), new element=w1105) -> (w1102:cluster{u32, u32}[])  [unwired: 1 in]
        n448 = local write "Master"(FALSE ("Master")) -> ()
        n449 = property on="Gluteos Bool" class="Bool"("Colors [4]"=w1103) -> ()  [unwired: 2 in, 2 out]
        n450 = Index Array(array=w1092) -> (element=w1098:cluster{u32, u32})  [unwired: 1 in]
        n451 = property on="Abdomen Bool" class="Bool"("Colors [4]"=w1102) -> ()  [unwired: 2 in, 2 out]
        n452 = property on="Lumbares Bool" class="Bool"("Colors [4]"=w1102) -> ()  [unwired: 2 in, 2 out]
        n453 = property on="Isquiotibiales Bool" class="Bool"("Colors [4]"=w1102) -> ()  [unwired: 2 in, 2 out]
        n454 = property on="Cuadriceps Bool" class="Bool"("Colors [4]"=w1102) -> ()  [unwired: 2 in, 2 out]
        n455 = Unbundle(w1098) -> (w1094:u32)  [unwired: 1 out]
        n456 = property on="Pectorales Bool" class="Bool"("Colors [4]"=w1102) -> ()  [unwired: 2 in, 2 out]
        n457 = property on="Dorsales Bool" class="Bool"("Colors [4]"=w1102) -> ()  [unwired: 2 in, 2 out]
        n458 = property on="Trapecio Bool" class="Bool"("Colors [4]"=w1102) -> ()  [unwired: 2 in, 2 out]
        n459 = property on="Opcional Bool" class="Bool"("Colors [4]"=w1102) -> ()  [unwired: 2 in, 2 out]
        n460 = property on="Biceps Bool" class="Bool"("Colors [4]"=w1102) -> ()  [unwired: 2 in, 2 out]
        n461 = Bundle(w1094, "Boolean Text.Text Colors:Text Color"=u32 40709) -> (w1097:T3)  [unwired: 1 in]
        n462 = Replace Array Subset(array=w1092, new element=w1097, index=0) -> (w1091:cluster{u32, u32}[])
        n463 = property on="Master" class="Bool (strict)"(error in=w1089, "Colors [4]"=w1091) -> (error out=w1090:errorcluster)  [unwired: 1 in, 1 out]
        n464 = property on="Master" class="Bool (strict)"(error in=w1090, "BoolText.TextColor"=u32 16448250 ("Boolean Text.Text Colors:Text Color")) -> ()  [unwired: 1 in, 2 out]
      }
      event "Abdomen Bool": Value Change {
        n465 = event-data() -> ()  [unwired: 1 in, 6 out]
        n466 = Bundle By Name(cluster=cluster{"Color Box":u32, "Color Box 2":u32} {"Color Box"=12369084, "Color Box 2"=12369084}, "Color Box"=u32 16711680 ("Color Box 2")) -> (w1134:cluster{"Color Box":u32, "Color Box 2":u32})
        n467 = Bundle By Name(cluster=cluster{"Color Box":u32, "Color Box 2":u32} {"Color Box"=12369084, "Color Box 2"=12369084}, "Color Box"=u32 12369084 ("Color Box 2")) -> (w1130:cluster{"Color Box":u32, "Color Box 2":u32})
        n468 = Bundle By Name(cluster=w1125, "Label"="Abdomen" ("Message")) -> (w1124:T2)
        n469 = property on="Master" class="Bool (strict)"() -> (error out=w1114:errorcluster, "Colors [4]"=w1117:cluster{u32, u32}[])  [unwired: 2 in, 1 out]
        n470 = Insert Into Array(array=cluster{u32, u32}[] [] ("Colors [4]"), new element=w1134) -> (w1128:cluster{u32, u32}[])  [unwired: 1 in]
        n471 = Insert Into Array(array=cluster{u32, u32}[] [] ("Colors [4]"), new element=w1130) -> (w1127:cluster{u32, u32}[])  [unwired: 1 in]
        n472 = property on="Abdomen Bool" class="Bool"("Colors [4]"=w1128) -> ()  [unwired: 2 in, 2 out]
        n473 = Index Array(array=w1117) -> (element=w1123:cluster{u32, u32})  [unwired: 1 in]
        n474 = local write "Master"(FALSE ("Master")) -> ()
        n475 = property on="Gluteos Bool" class="Bool"("Colors [4]"=w1127) -> ()  [unwired: 2 in, 2 out]
        n476 = property on="Lumbares Bool" class="Bool"("Colors [4]"=w1127) -> ()  [unwired: 2 in, 2 out]
        n477 = property on="Isquiotibiales Bool" class="Bool"("Colors [4]"=w1127) -> ()  [unwired: 2 in, 2 out]
        n478 = property on="Cuadriceps Bool" class="Bool"("Colors [4]"=w1127) -> ()  [unwired: 2 in, 2 out]
        n479 = Unbundle(w1123) -> (w1119:u32)  [unwired: 1 out]
        n480 = property on="Pectorales Bool" class="Bool"("Colors [4]"=w1127) -> ()  [unwired: 2 in, 2 out]
        n481 = property on="Dorsales Bool" class="Bool"("Colors [4]"=w1127) -> ()  [unwired: 2 in, 2 out]
        n482 = property on="Trapecio Bool" class="Bool"("Colors [4]"=w1127) -> ()  [unwired: 2 in, 2 out]
        n483 = property on="Opcional Bool" class="Bool"("Colors [4]"=w1127) -> ()  [unwired: 2 in, 2 out]
        n484 = property on="Biceps Bool" class="Bool"("Colors [4]"=w1127) -> ()  [unwired: 2 in, 2 out]
        n485 = Bundle(w1119, "Boolean Text.Text Colors:Text Color"=u32 40709) -> (w1122:T3)  [unwired: 1 in]
        n486 = Replace Array Subset(array=w1117, new element=w1122, index=0) -> (w1116:cluster{u32, u32}[])
        n487 = property on="Master" class="Bool (strict)"(error in=w1114, "Colors [4]"=w1116) -> (error out=w1115:errorcluster)  [unwired: 1 in, 1 out]
        n488 = property on="Master" class="Bool (strict)"(error in=w1115, "BoolText.TextColor"=u32 16448250 ("Boolean Text.Text Colors:Text Color")) -> ()  [unwired: 1 in, 2 out]
      }
      event "Lumbares Bool": Value Change {
        n489 = event-data() -> ()  [unwired: 1 in, 6 out]
        n490 = Bundle By Name(cluster=cluster{"Color Box":u32, "Color Box 2":u32} {"Color Box"=12369084, "Color Box 2"=12369084}, "Color Box"=u32 16711680 ("Color Box 2")) -> (w1159:cluster{"Color Box":u32, "Color Box 2":u32})
        n491 = Bundle By Name(cluster=cluster{"Color Box":u32, "Color Box 2":u32} {"Color Box"=12369084, "Color Box 2"=12369084}, "Color Box"=u32 12369084 ("Color Box 2")) -> (w1155:cluster{"Color Box":u32, "Color Box 2":u32})
        n492 = property on="Master" class="Bool (strict)"() -> (error out=w1139:errorcluster, "Colors [4]"=w1142:cluster{u32, u32}[])  [unwired: 2 in, 1 out]
        n493 = Insert Into Array(array=cluster{u32, u32}[] [] ("Colors [4]"), new element=w1159) -> (w1153:cluster{u32, u32}[])  [unwired: 1 in]
        n494 = Insert Into Array(array=cluster{u32, u32}[] [] ("Colors [4]"), new element=w1155) -> (w1152:cluster{u32, u32}[])  [unwired: 1 in]
        n495 = Bundle By Name(cluster=w1150, "Label"="Lumbares" ("Message")) -> (w1149:T2)
        n496 = property on="Lumbares Bool" class="Bool"("Colors [4]"=w1153) -> ()  [unwired: 2 in, 2 out]
        n497 = local write "Master"(FALSE ("Master")) -> ()
        n498 = Index Array(array=w1142) -> (element=w1148:cluster{u32, u32})  [unwired: 1 in]
        n499 = property on="Gluteos Bool" class="Bool"("Colors [4]"=w1152) -> ()  [unwired: 2 in, 2 out]
        n500 = property on="Abdomen Bool" class="Bool"("Colors [4]"=w1152) -> ()  [unwired: 2 in, 2 out]
        n501 = property on="Isquiotibiales Bool" class="Bool"("Colors [4]"=w1152) -> ()  [unwired: 2 in, 2 out]
        n502 = property on="Cuadriceps Bool" class="Bool"("Colors [4]"=w1152) -> ()  [unwired: 2 in, 2 out]
        n503 = Unbundle(w1148) -> (w1144:u32)  [unwired: 1 out]
        n504 = property on="Pectorales Bool" class="Bool"("Colors [4]"=w1152) -> ()  [unwired: 2 in, 2 out]
        n505 = property on="Dorsales Bool" class="Bool"("Colors [4]"=w1152) -> ()  [unwired: 2 in, 2 out]
        n506 = property on="Trapecio Bool" class="Bool"("Colors [4]"=w1152) -> ()  [unwired: 2 in, 2 out]
        n507 = property on="Opcional Bool" class="Bool"("Colors [4]"=w1152) -> ()  [unwired: 2 in, 2 out]
        n508 = property on="Biceps Bool" class="Bool"("Colors [4]"=w1152) -> ()  [unwired: 2 in, 2 out]
        n509 = Bundle(w1144, "Boolean Text.Text Colors:Text Color"=u32 40709) -> (w1147:T3)  [unwired: 1 in]
        n510 = Replace Array Subset(array=w1142, new element=w1147, index=0) -> (w1141:cluster{u32, u32}[])
        n511 = property on="Master" class="Bool (strict)"(error in=w1139, "Colors [4]"=w1141) -> (error out=w1140:errorcluster)  [unwired: 1 in, 1 out]
        n512 = property on="Master" class="Bool (strict)"(error in=w1140, "BoolText.TextColor"=u32 16448250 ("Boolean Text.Text Colors:Text Color")) -> ()  [unwired: 1 in, 2 out]
      }
      event "Dorsales Bool": Value Change {
        n513 = event-data() -> ()  [unwired: 1 in, 6 out]
        n514 = Bundle By Name(cluster=cluster{"Color Box":u32, "Color Box 2":u32} {"Color Box"=12369084, "Color Box 2"=12369084}, "Color Box"=u32 16711680 ("Color Box 2")) -> (w1184:cluster{"Color Box":u32, "Color Box 2":u32})
        n515 = Bundle By Name(cluster=cluster{"Color Box":u32, "Color Box 2":u32} {"Color Box"=12369084, "Color Box 2"=12369084}, "Color Box"=u32 12369084 ("Color Box 2")) -> (w1180:cluster{"Color Box":u32, "Color Box 2":u32})
        n516 = property on="Master" class="Bool (strict)"() -> (error out=w1164:errorcluster, "Colors [4]"=w1167:cluster{u32, u32}[])  [unwired: 2 in, 1 out]
        n517 = Bundle By Name(cluster=w1175, "Label"="Dorsales" ("Message")) -> (w1174:T2)
        n518 = Insert Into Array(array=cluster{u32, u32}[] [] ("Colors [4]"), new element=w1184) -> (w1177:cluster{u32, u32}[])  [unwired: 1 in]
        n519 = Insert Into Array(array=cluster{u32, u32}[] [] ("Colors [4]"), new element=w1180) -> (w1178:cluster{u32, u32}[])  [unwired: 1 in]
        n520 = Index Array(array=w1167) -> (element=w1173:cluster{u32, u32})  [unwired: 1 in]
        n521 = local write "Master"(FALSE ("Master")) -> ()
        n522 = property on="Gluteos Bool" class="Bool"("Colors [4]"=w1178) -> ()  [unwired: 2 in, 2 out]
        n523 = property on="Abdomen Bool" class="Bool"("Colors [4]"=w1178) -> ()  [unwired: 2 in, 2 out]
        n524 = Unbundle(w1173) -> (w1169:u32)  [unwired: 1 out]
        n525 = property on="Isquiotibiales Bool" class="Bool"("Colors [4]"=w1178) -> ()  [unwired: 2 in, 2 out]
        n526 = property on="Cuadriceps Bool" class="Bool"("Colors [4]"=w1178) -> ()  [unwired: 2 in, 2 out]
        n527 = property on="Dorsales Bool" class="Bool"("Colors [4]"=w1177) -> ()  [unwired: 2 in, 2 out]
        n528 = Bundle(w1169, "Boolean Text.Text Colors:Text Color"=u32 40709) -> (w1172:T3)  [unwired: 1 in]
        n529 = property on="Pectorales Bool" class="Bool"("Colors [4]"=w1178) -> ()  [unwired: 2 in, 2 out]
        n530 = property on="Lumbares Bool" class="Bool"("Colors [4]"=w1178) -> ()  [unwired: 2 in, 2 out]
        n531 = property on="Trapecio Bool" class="Bool"("Colors [4]"=w1178) -> ()  [unwired: 2 in, 2 out]
        n532 = property on="Opcional Bool" class="Bool"("Colors [4]"=w1178) -> ()  [unwired: 2 in, 2 out]
        n533 = property on="Biceps Bool" class="Bool"("Colors [4]"=w1178) -> ()  [unwired: 2 in, 2 out]
        n534 = Replace Array Subset(array=w1167, new element=w1172, index=0) -> (w1166:cluster{u32, u32}[])
        n535 = property on="Master" class="Bool (strict)"(error in=w1164, "Colors [4]"=w1166) -> (error out=w1165:errorcluster)  [unwired: 1 in, 1 out]
        n536 = property on="Master" class="Bool (strict)"(error in=w1165, "BoolText.TextColor"=u32 16448250 ("Boolean Text.Text Colors:Text Color")) -> ()  [unwired: 1 in, 2 out]
      }
      event "Trapecio Bool": Value Change {
        n537 = event-data() -> ()  [unwired: 1 in, 6 out]
        n538 = Bundle By Name(cluster=cluster{"Color Box":u32, "Color Box 2":u32} {"Color Box"=12369084, "Color Box 2"=12369084}, "Color Box"=u32 16711680 ("Color Box 2")) -> (w1209:cluster{"Color Box":u32, "Color Box 2":u32})
        n539 = Bundle By Name(cluster=cluster{"Color Box":u32, "Color Box 2":u32} {"Color Box"=12369084, "Color Box 2"=12369084}, "Color Box"=u32 12369084 ("Color Box 2")) -> (w1205:cluster{"Color Box":u32, "Color Box 2":u32})
        n540 = Bundle By Name(cluster=w1200, "Label"="Trapecio" ("Message")) -> (w1199:T2)
        n541 = property on="Master" class="Bool (strict)"() -> (error out=w1189:errorcluster, "Colors [4]"=w1192:cluster{u32, u32}[])  [unwired: 2 in, 1 out]
        n542 = Insert Into Array(array=cluster{u32, u32}[] [] ("Colors [4]"), new element=w1209) -> (w1202:cluster{u32, u32}[])  [unwired: 1 in]
        n543 = Insert Into Array(array=cluster{u32, u32}[] [] ("Colors [4]"), new element=w1205) -> (w1203:cluster{u32, u32}[])  [unwired: 1 in]
        n544 = local write "Master"(FALSE ("Master")) -> ()
        n545 = property on="Trapecio Bool" class="Bool"("Colors [4]"=w1202) -> ()  [unwired: 2 in, 2 out]
        n546 = property on="Gluteos Bool" class="Bool"("Colors [4]"=w1203) -> ()  [unwired: 2 in, 2 out]
        n547 = property on="Abdomen Bool" class="Bool"("Colors [4]"=w1203) -> ()  [unwired: 2 in, 2 out]
        n548 = Index Array(array=w1192) -> (element=w1198:cluster{u32, u32})  [unwired: 1 in]
        n549 = property on="Isquiotibiales Bool" class="Bool"("Colors [4]"=w1203) -> ()  [unwired: 2 in, 2 out]
        n550 = property on="Cuadriceps Bool" class="Bool"("Colors [4]"=w1203) -> ()  [unwired: 2 in, 2 out]
        n551 = Unbundle(w1198) -> (w1194:u32)  [unwired: 1 out]
        n552 = property on="Pectorales Bool" class="Bool"("Colors [4]"=w1203) -> ()  [unwired: 2 in, 2 out]
        n553 = property on="Lumbares Bool" class="Bool"("Colors [4]"=w1203) -> ()  [unwired: 2 in, 2 out]
        n554 = property on="Dorsales Bool" class="Bool"("Colors [4]"=w1203) -> ()  [unwired: 2 in, 2 out]
        n555 = property on="Opcional Bool" class="Bool"("Colors [4]"=w1203) -> ()  [unwired: 2 in, 2 out]
        n556 = property on="Biceps Bool" class="Bool"("Colors [4]"=w1203) -> ()  [unwired: 2 in, 2 out]
        n557 = Bundle(w1194, "Boolean Text.Text Colors:Text Color"=u32 40709) -> (w1197:T3)  [unwired: 1 in]
        n558 = Replace Array Subset(array=w1192, new element=w1197, index=0) -> (w1191:cluster{u32, u32}[])
        n559 = property on="Master" class="Bool (strict)"(error in=w1189, "Colors [4]"=w1191) -> (error out=w1190:errorcluster)  [unwired: 1 in, 1 out]
        n560 = property on="Master" class="Bool (strict)"(error in=w1190, "BoolText.TextColor"=u32 16448250 ("Boolean Text.Text Colors:Text Color")) -> ()  [unwired: 1 in, 2 out]
      }
      event "Pectorales Bool": Value Change {
        n561 = event-data() -> ()  [unwired: 1 in, 6 out]
        n562 = Bundle By Name(cluster=cluster{"Color Box":u32, "Color Box 2":u32} {"Color Box"=12369084, "Color Box 2"=12369084}, "Color Box"=u32 16711680 ("Color Box 2")) -> (w1234:cluster{"Color Box":u32, "Color Box 2":u32})
        n563 = Bundle By Name(cluster=cluster{"Color Box":u32, "Color Box 2":u32} {"Color Box"=12369084, "Color Box 2"=12369084}, "Color Box"=u32 12369084 ("Color Box 2")) -> (w1230:cluster{"Color Box":u32, "Color Box 2":u32})
        n564 = property on="Master" class="Bool (strict)"() -> (error out=w1214:errorcluster, "Colors [4]"=w1217:cluster{u32, u32}[])  [unwired: 2 in, 1 out]
        n565 = Bundle By Name(cluster=w1225, "Label"="Pectorales" ("Message")) -> (w1224:T2)
        n566 = Insert Into Array(array=cluster{u32, u32}[] [] ("Colors [4]"), new element=w1234) -> (w1227:cluster{u32, u32}[])  [unwired: 1 in]
        n567 = Insert Into Array(array=cluster{u32, u32}[] [] ("Colors [4]"), new element=w1230) -> (w1228:cluster{u32, u32}[])  [unwired: 1 in]
        n568 = local write "Master"(FALSE ("Master")) -> ()
        n569 = Index Array(array=w1217) -> (element=w1223:cluster{u32, u32})  [unwired: 1 in]
        n570 = Unbundle(w1223) -> (w1219:u32)  [unwired: 1 out]
        n571 = property on="Pectorales Bool" class="Bool"("Colors [4]"=w1227) -> ()  [unwired: 2 in, 2 out]
        n572 = property on="Gluteos Bool" class="Bool"("Colors [4]"=w1228) -> ()  [unwired: 2 in, 2 out]
        n573 = property on="Abdomen Bool" class="Bool"("Colors [4]"=w1228) -> ()  [unwired: 2 in, 2 out]
        n574 = property on="Isquiotibiales Bool" class="Bool"("Colors [4]"=w1228) -> ()  [unwired: 2 in, 2 out]
        n575 = property on="Cuadriceps Bool" class="Bool"("Colors [4]"=w1228) -> ()  [unwired: 2 in, 2 out]
        n576 = Bundle(w1219, "Boolean Text.Text Colors:Text Color"=u32 40709) -> (w1222:T3)  [unwired: 1 in]
        n577 = property on="Trapecio Bool" class="Bool"("Colors [4]"=w1228) -> ()  [unwired: 2 in, 2 out]
        n578 = property on="Lumbares Bool" class="Bool"("Colors [4]"=w1228) -> ()  [unwired: 2 in, 2 out]
        n579 = property on="Dorsales Bool" class="Bool"("Colors [4]"=w1228) -> ()  [unwired: 2 in, 2 out]
        n580 = property on="Opcional Bool" class="Bool"("Colors [4]"=w1228) -> ()  [unwired: 2 in, 2 out]
        n581 = property on="Biceps Bool" class="Bool"("Colors [4]"=w1228) -> ()  [unwired: 2 in, 2 out]
        n582 = Replace Array Subset(array=w1217, new element=w1222, index=0) -> (w1216:cluster{u32, u32}[])
        n583 = property on="Master" class="Bool (strict)"(error in=w1214, "Colors [4]"=w1216) -> (error out=w1215:errorcluster)  [unwired: 1 in, 1 out]
        n584 = property on="Master" class="Bool (strict)"(error in=w1215, "BoolText.TextColor"=u32 16448250 ("Boolean Text.Text Colors:Text Color")) -> ()  [unwired: 1 in, 2 out]
      }
      event "Biceps Bool": Value Change {
        n585 = event-data() -> ()  [unwired: 1 in, 6 out]
        n586 = Bundle By Name(cluster=cluster{"Color Box":u32, "Color Box 2":u32} {"Color Box"=12369084, "Color Box 2"=12369084}, "Color Box"=u32 16711680 ("Color Box 2")) -> (w1259:cluster{"Color Box":u32, "Color Box 2":u32})
        n587 = Bundle By Name(cluster=cluster{"Color Box":u32, "Color Box 2":u32} {"Color Box"=12369084, "Color Box 2"=12369084}, "Color Box"=u32 12369084 ("Color Box 2")) -> (w1255:cluster{"Color Box":u32, "Color Box 2":u32})
        n588 = property on="Master" class="Bool (strict)"() -> (error out=w1239:errorcluster, "Colors [4]"=w1242:cluster{u32, u32}[])  [unwired: 2 in, 1 out]
        n589 = Bundle By Name(cluster=w1250, "Label"="Biceps" ("Message")) -> (w1249:T2)
        n590 = Insert Into Array(array=cluster{u32, u32}[] [] ("Colors [4]"), new element=w1259) -> (w1252:cluster{u32, u32}[])  [unwired: 1 in]
        n591 = Insert Into Array(array=cluster{u32, u32}[] [] ("Colors [4]"), new element=w1255) -> (w1253:cluster{u32, u32}[])  [unwired: 1 in]
        n592 = Index Array(array=w1242) -> (element=w1248:cluster{u32, u32})  [unwired: 1 in]
        n593 = local write "Master"(FALSE ("Master")) -> ()
        n594 = Unbundle(w1248) -> (w1244:u32)  [unwired: 1 out]
        n595 = property on="Biceps Bool" class="Bool"("Colors [4]"=w1252) -> ()  [unwired: 2 in, 2 out]
        n596 = property on="Gluteos Bool" class="Bool"("Colors [4]"=w1253) -> ()  [unwired: 2 in, 2 out]
        n597 = property on="Abdomen Bool" class="Bool"("Colors [4]"=w1253) -> ()  [unwired: 2 in, 2 out]
        n598 = property on="Isquiotibiales Bool" class="Bool"("Colors [4]"=w1253) -> ()  [unwired: 2 in, 2 out]
        n599 = property on="Cuadriceps Bool" class="Bool"("Colors [4]"=w1253) -> ()  [unwired: 2 in, 2 out]
        n600 = Bundle(w1244, "Boolean Text.Text Colors:Text Color"=u32 40709) -> (w1247:T3)  [unwired: 1 in]
        n601 = property on="Trapecio Bool" class="Bool"("Colors [4]"=w1253) -> ()  [unwired: 2 in, 2 out]
        n602 = property on="Lumbares Bool" class="Bool"("Colors [4]"=w1253) -> ()  [unwired: 2 in, 2 out]
        n603 = property on="Dorsales Bool" class="Bool"("Colors [4]"=w1253) -> ()  [unwired: 2 in, 2 out]
        n604 = property on="Opcional Bool" class="Bool"("Colors [4]"=w1253) -> ()  [unwired: 2 in, 2 out]
        n605 = property on="Pectorales Bool" class="Bool"("Colors [4]"=w1253) -> ()  [unwired: 2 in, 2 out]
        n606 = Replace Array Subset(array=w1242, new element=w1247, index=0) -> (w1241:cluster{u32, u32}[])
        n607 = property on="Master" class="Bool (strict)"(error in=w1239, "Colors [4]"=w1241) -> (error out=w1240:errorcluster)  [unwired: 1 in, 1 out]
        n608 = property on="Master" class="Bool (strict)"(error in=w1240, "BoolText.TextColor"=u32 16448250 ("Boolean Text.Text Colors:Text Color")) -> ()  [unwired: 1 in, 2 out]
      }
      event "Opcional Bool": Value Change {
        n609 = event-data() -> ()  [unwired: 1 in, 6 out]
        n610 = Bundle By Name(cluster=cluster{"Color Box":u32, "Color Box 2":u32} {"Color Box"=12369084, "Color Box 2"=12369084}, "Color Box"=u32 16711680 ("Color Box 2")) -> (w1284:cluster{"Color Box":u32, "Color Box 2":u32})
        n611 = Bundle By Name(cluster=cluster{"Color Box":u32, "Color Box 2":u32} {"Color Box"=12369084, "Color Box 2"=12369084}, "Color Box"=u32 12369084 ("Color Box 2")) -> (w1280:cluster{"Color Box":u32, "Color Box 2":u32})
        n612 = property on="Master" class="Bool (strict)"() -> (error out=w1264:errorcluster, "Colors [4]"=w1267:cluster{u32, u32}[])  [unwired: 2 in, 1 out]
        n613 = Bundle By Name(cluster=w1275, "Label"="Opcional" ("Message")) -> (w1274:T2)
        n614 = Insert Into Array(array=cluster{u32, u32}[] [] ("Colors [4]"), new element=w1284) -> (w1277:cluster{u32, u32}[])  [unwired: 1 in]
        n615 = Insert Into Array(array=cluster{u32, u32}[] [] ("Colors [4]"), new element=w1280) -> (w1278:cluster{u32, u32}[])  [unwired: 1 in]
        n616 = Index Array(array=w1267) -> (element=w1273:cluster{u32, u32})  [unwired: 1 in]
        n617 = local write "Master"(FALSE ("Master")) -> ()
        n618 = property on="Opcional Bool" class="Bool"("Colors [4]"=w1277) -> ()  [unwired: 2 in, 2 out]
        n619 = Unbundle(w1273) -> (w1269:u32)  [unwired: 1 out]
        n620 = property on="Gluteos Bool" class="Bool"("Colors [4]"=w1278) -> ()  [unwired: 2 in, 2 out]
        n621 = property on="Abdomen Bool" class="Bool"("Colors [4]"=w1278) -> ()  [unwired: 2 in, 2 out]
        n622 = property on="Isquiotibiales Bool" class="Bool"("Colors [4]"=w1278) -> ()  [unwired: 2 in, 2 out]
        n623 = property on="Cuadriceps Bool" class="Bool"("Colors [4]"=w1278) -> ()  [unwired: 2 in, 2 out]
        n624 = Bundle(w1269, "Boolean Text.Text Colors:Text Color"=u32 40709) -> (w1272:T3)  [unwired: 1 in]
        n625 = property on="Trapecio Bool" class="Bool"("Colors [4]"=w1278) -> ()  [unwired: 2 in, 2 out]
        n626 = property on="Lumbares Bool" class="Bool"("Colors [4]"=w1278) -> ()  [unwired: 2 in, 2 out]
        n627 = property on="Dorsales Bool" class="Bool"("Colors [4]"=w1278) -> ()  [unwired: 2 in, 2 out]
        n628 = property on="Biceps Bool" class="Bool"("Colors [4]"=w1278) -> ()  [unwired: 2 in, 2 out]
        n629 = property on="Pectorales Bool" class="Bool"("Colors [4]"=w1278) -> ()  [unwired: 2 in, 2 out]
        n630 = Replace Array Subset(array=w1267, new element=w1272, index=0) -> (w1266:cluster{u32, u32}[])
        n631 = property on="Master" class="Bool (strict)"(error in=w1264, "Colors [4]"=w1266) -> (error out=w1265:errorcluster)  [unwired: 1 in, 1 out]
        n632 = property on="Master" class="Bool (strict)"(error in=w1265, "BoolText.TextColor"=u32 16448250 ("Boolean Text.Text Colors:Text Color")) -> ()  [unwired: 1 in, 2 out]
      }
      event "Add Button": Value Change {
        n633 = event-data() -> ()  [unwired: 1 in, 6 out]
        n634 = Unbundle By Name(w1291) -> ("Label"=w1290:string)
        n635 = case shown="\"Cuadriceps\"" w1290 {
          tunnel: [w1294 w1309 w1322 w1332 w1345 w1358 w1371 w1384 w1397 w1410 w1423 w1436] -> w1292
          tunnel: w1291 -> [w1305 w1318 w1331 w1344 w1357 w1370 w1383 w1396 w1409 w1422 w1435 w1436]
          tunnel: w1289 -> [w1296 w1308 w1321 w1333 w1347 w1360 w1372 w1386 w1399 w1412 w1425 _]
          tunnel: w1288 -> [w1295 w1307 w1320 w1334 w1346 w1359 w1373 w1385 w1398 w1411 w1424 _]
          frame "Cuadriceps" {
            n636 = Unbundle By Name(w1305) -> ("Cuadriceps"=w1297:i32)
            n637 = Greater Or Equal To 0?(x=w1297) -> (x >= 0?=w1302:bool)
            n638 = Less Or Equal?(x=w1297, y=100) -> (x <= y?=w1300:bool)
            n639 = Add(x=w1297, y=5) -> (x+y=w1304:i32)
            n640 = And(x=w1302, y=w1300) -> (x .and. y?=w1301:bool)
            n641 = Select(t=w1304, s=w1301, f=w1297) -> (s? t:f=w1298:i32)
            n642 = Bundle By Name(cluster=w1305, "Cuadriceps"=w1298, "Label"="Cuadriceps") -> (w1294:T2)
            n643 = Enqueue Element At Opposite End(queue=w1295, element=w1294, error in (no error)=w1296) -> ()  [unwired: 1 in, 3 out]
          }
          frame "Isquiotibiales" {
            n644 = Unbundle By Name(w1318) -> ("Isquiotibiales"=w1310:i32)
            n645 = Greater Or Equal To 0?(x=w1310) -> (x >= 0?=w1315:bool)
            n646 = Less Or Equal?(x=w1310, y=100) -> (x <= y?=w1313:bool)
            n647 = Add(x=w1310, y=5) -> (x+y=w1317:i32)
            n648 = And(x=w1315, y=w1313) -> (x .and. y?=w1314:bool)
            n649 = Select(t=w1317, s=w1314, f=w1310) -> (s? t:f=w1311:i32)
            n650 = Bundle By Name(cluster=w1318, "Isquiotibiales"=w1311, "Label"="Isquiotibiales") -> (w1309:T2)
            n651 = Enqueue Element At Opposite End(queue=w1307, element=w1309, error in (no error)=w1308) -> ()  [unwired: 1 in, 3 out]
          }
          frame "Gluteos" {
            n652 = Unbundle By Name(w1331) -> ("Gluteos"=w1323:i32)
            n653 = Greater Or Equal To 0?(x=w1323) -> (x >= 0?=w1328:bool)
            n654 = Less Or Equal?(x=w1323, y=100) -> (x <= y?=w1326:bool)
            n655 = Add(x=w1323, y=5) -> (x+y=w1330:i32)
            n656 = And(x=w1328, y=w1326) -> (x .and. y?=w1327:bool)
            n657 = Select(t=w1330, s=w1327, f=w1323) -> (s? t:f=w1324:i32)
            n658 = Bundle By Name(cluster=w1331, "Gluteos"=w1324, "Label"="Gluteos") -> (w1322:T2)
            n659 = Enqueue Element At Opposite End(queue=w1320, element=w1322, error in (no error)=w1321) -> ()  [unwired: 1 in, 3 out]
          }
          frame "Abdomen" {
            n660 = Unbundle By Name(w1344) -> ("Abdomen"=w1336:i32)
            n661 = Greater Or Equal To 0?(x=w1336) -> (x >= 0?=w1341:bool)
            n662 = Less Or Equal?(x=w1336, y=100) -> (x <= y?=w1339:bool)
            n663 = Add(x=w1336, y=5) -> (x+y=w1343:i32)
            n664 = And(x=w1341, y=w1339) -> (x .and. y?=w1340:bool)
            n665 = Select(t=w1343, s=w1340, f=w1336) -> (s? t:f=w1337:i32)
            n666 = Bundle By Name(cluster=w1344, "Abdomen"=w1337, "Label"="Abdomen") -> (w1332:T2)
            n667 = Enqueue Element At Opposite End(queue=w1334, element=w1332, error in (no error)=w1333) -> ()  [unwired: 1 in, 3 out]
          }
          frame "Lumbares" {
            n668 = Unbundle By Name(w1357) -> ("Lumbares"=w1349:i32)
            n669 = Greater Or Equal To 0?(x=w1349) -> (x >= 0?=w1354:bool)
            n670 = Less Or Equal?(x=w1349, y=100) -> (x <= y?=w1352:bool)
            n671 = Add(x=w1349, y=5) -> (x+y=w1356:i32)
            n672 = And(x=w1354, y=w1352) -> (x .and. y?=w1353:bool)
            n673 = Select(t=w1356, s=w1353, f=w1349) -> (s? t:f=w1350:i32)
            n674 = Bundle By Name(cluster=w1357, "Lumbares"=w1350, "Label"="Lumbares") -> (w1345:T2)
            n675 = Enqueue Element At Opposite End(queue=w1346, element=w1345, error in (no error)=w1347) -> ()  [unwired: 1 in, 3 out]
          }
          frame "Dorsales" {
            n676 = Unbundle By Name(w1370) -> ("Dorsales"=w1362:i32)
            n677 = Greater Or Equal To 0?(x=w1362) -> (x >= 0?=w1367:bool)
            n678 = Less Or Equal?(x=w1362, y=100) -> (x <= y?=w1365:bool)
            n679 = Add(x=w1362, y=5) -> (x+y=w1369:i32)
            n680 = And(x=w1367, y=w1365) -> (x .and. y?=w1366:bool)
            n681 = Select(t=w1369, s=w1366, f=w1362) -> (s? t:f=w1363:i32)
            n682 = Bundle By Name(cluster=w1370, "Dorsales"=w1363, "Label"="Dorsales") -> (w1358:T2)
            n683 = Enqueue Element At Opposite End(queue=w1359, element=w1358, error in (no error)=w1360) -> ()  [unwired: 1 in, 3 out]
          }
          frame "Trapecio" {
            n684 = Unbundle By Name(w1383) -> ("Trapecio"=w1375:i32)
            n685 = Greater Or Equal To 0?(x=w1375) -> (x >= 0?=w1380:bool)
            n686 = Less Or Equal?(x=w1375, y=100) -> (x <= y?=w1378:bool)
            n687 = Add(x=w1375, y=5) -> (x+y=w1382:i32)
            n688 = And(x=w1380, y=w1378) -> (x .and. y?=w1379:bool)
            n689 = Select(t=w1382, s=w1379, f=w1375) -> (s? t:f=w1376:i32)
            n690 = Bundle By Name(cluster=w1383, "Trapecio"=w1376, "Label"="Trapecio") -> (w1371:T2)
            n691 = Enqueue Element At Opposite End(queue=w1373, element=w1371, error in (no error)=w1372) -> ()  [unwired: 1 in, 3 out]
          }
          frame "Pectorales" {
            n692 = Unbundle By Name(w1396) -> ("Pectorales"=w1388:i32)
            n693 = Greater Or Equal To 0?(x=w1388) -> (x >= 0?=w1393:bool)
            n694 = Less Or Equal?(x=w1388, y=100) -> (x <= y?=w1391:bool)
            n695 = Add(x=w1388, y=5) -> (x+y=w1395:i32)
            n696 = And(x=w1393, y=w1391) -> (x .and. y?=w1392:bool)
            n697 = Select(t=w1395, s=w1392, f=w1388) -> (s? t:f=w1389:i32)
            n698 = Bundle By Name(cluster=w1396, "Pectorales"=w1389, "Label"="Pectorales") -> (w1384:T2)
            n699 = Enqueue Element At Opposite End(queue=w1385, element=w1384, error in (no error)=w1386) -> ()  [unwired: 1 in, 3 out]
          }
          frame "Biceps" {
            n700 = Unbundle By Name(w1409) -> ("Biceps"=w1401:i32)
            n701 = Greater Or Equal To 0?(x=w1401) -> (x >= 0?=w1406:bool)
            n702 = Less Or Equal?(x=w1401, y=100) -> (x <= y?=w1404:bool)
            n703 = Add(x=w1401, y=5) -> (x+y=w1408:i32)
            n704 = And(x=w1406, y=w1404) -> (x .and. y?=w1405:bool)
            n705 = Select(t=w1408, s=w1405, f=w1401) -> (s? t:f=w1402:i32)
            n706 = Bundle By Name(cluster=w1409, "Biceps"=w1402, "Label"="Biceps") -> (w1397:T2)
            n707 = Enqueue Element At Opposite End(queue=w1398, element=w1397, error in (no error)=w1399) -> ()  [unwired: 1 in, 3 out]
          }
          frame "Opcional" {
            n708 = Unbundle By Name(w1422) -> ("Opcional"=w1414:i32)
            n709 = Greater Or Equal To 0?(x=w1414) -> (x >= 0?=w1419:bool)
            n710 = Less Or Equal?(x=w1414, y=100) -> (x <= y?=w1417:bool)
            n711 = Add(x=w1414, y=5) -> (x+y=w1421:i32)
            n712 = And(x=w1419, y=w1417) -> (x .and. y?=w1418:bool)
            n713 = Select(t=w1421, s=w1418, f=w1414) -> (s? t:f=w1415:i32)
            n714 = Bundle By Name(cluster=w1422, "Opcional"=w1415, "Label"="Opcional") -> (w1410:T2)
            n715 = Enqueue Element At Opposite End(queue=w1411, element=w1410, error in (no error)=w1412) -> ()  [unwired: 1 in, 3 out]
          }
          frame "Master" {
            n716 = Unbundle By Name(w1435) -> ("Master"=w1427:i32)
            n717 = Greater Or Equal To 0?(x=w1427) -> (x >= 0?=w1432:bool)
            n718 = Less?(x=w1427, y=100) -> (x < y?=w1430:bool)
            n719 = Add(x=w1427, y=5) -> (x+y=w1434:i32)
            n720 = And(x=w1432, y=w1430) -> (x .and. y?=w1431:bool)
            n721 = Select(t=w1434, s=w1431, f=w1427) -> (s? t:f=w1428:i32)
            n722 = Bundle By Name(cluster=w1435, "Master"=w1428, "Label"="Master") -> (w1423:T2)
            n723 = Enqueue Element At Opposite End(queue=w1424, element=w1423, error in (no error)=w1425) -> ()  [unwired: 1 in, 3 out]
          }
          frame Default {
          }
        }
      }
      event "Remove Button": Value Change {
        n724 = event-data() -> ()  [unwired: 1 in, 6 out]
        n725 = Unbundle By Name(w1440) -> ("Label"=w1439:string)
        n726 = case shown="\"Cuadriceps\"" w1439 {
          tunnel: [w1442 w1453 w1462 w1472 w1482 w1492 w1503 w1512 w1522 w1532 w1542 w1552] -> w1441
          tunnel: w1440 -> [w1451 w1461 w1471 w1481 w1491 w1501 w1511 w1521 w1531 w1541 w1551 w1552]
          tunnel: w1438 -> [w1443 w1454 w1463 w1473 w1484 w1493 w1505 w1513 w1524 w1534 w1544 _]
          tunnel: w1437 -> [w1444 w1455 w1464 w1474 w1483 w1494 w1504 w1514 w1523 w1533 w1543 _]
          frame "Cuadriceps" {
            n727 = Unbundle By Name(w1451) -> ("Cuadriceps"=w1446:i32)
            n728 = Greater Than 0?(x=w1446) -> (x > 0?=w1448:bool)
            n729 = Subtract(x=w1446, y=5) -> (x-y=w1449:i32)
            n730 = Select(t=w1449, s=w1448, f=w1446) -> (s? t:f=w1447:i32)
            n731 = Bundle By Name(cluster=w1451, "Cuadriceps"=w1447, "Label"="Cuadriceps") -> (w1442:T2)
            n732 = Enqueue Element At Opposite End(queue=w1443, element=w1442, error in (no error)=w1444) -> ()  [unwired: 1 in, 3 out]
          }
          frame "Isquiotibiales" {
            n733 = Unbundle By Name(w1461) -> ("Isquiotibiales"=w1456:i32)
            n734 = Greater Than 0?(x=w1456) -> (x > 0?=w1458:bool)
            n735 = Subtract(x=w1456, y=5) -> (x-y=w1459:i32)
            n736 = Select(t=w1459, s=w1458, f=w1456) -> (s? t:f=w1457:i32)
            n737 = Bundle By Name(cluster=w1461, "Isquiotibiales"=w1457, "Label"="Isquiotibiales") -> (w1453:T2)
            n738 = Enqueue Element At Opposite End(queue=w1454, element=w1453, error in (no error)=w1455) -> ()  [unwired: 1 in, 3 out]
          }
          frame "Gluteos" {
            n739 = Unbundle By Name(w1471) -> ("Gluteos"=w1466:i32)
            n740 = Greater Than 0?(x=w1466) -> (x > 0?=w1468:bool)
            n741 = Subtract(x=w1466, y=5) -> (x-y=w1469:i32)
            n742 = Select(t=w1469, s=w1468, f=w1466) -> (s? t:f=w1467:i32)
            n743 = Bundle By Name(cluster=w1471, "Gluteos"=w1467, "Label"="Gluteos") -> (w1462:T2)
            n744 = Enqueue Element At Opposite End(queue=w1463, element=w1462, error in (no error)=w1464) -> ()  [unwired: 1 in, 3 out]
          }
          frame "Abdomen" {
            n745 = Unbundle By Name(w1481) -> ("Abdomen"=w1476:i32)
            n746 = Greater Than 0?(x=w1476) -> (x > 0?=w1478:bool)
            n747 = Subtract(x=w1476, y=5) -> (x-y=w1479:i32)
            n748 = Select(t=w1479, s=w1478, f=w1476) -> (s? t:f=w1477:i32)
            n749 = Bundle By Name(cluster=w1481, "Abdomen"=w1477, "Label"="Abdomen") -> (w1472:T2)
            n750 = Enqueue Element At Opposite End(queue=w1473, element=w1472, error in (no error)=w1474) -> ()  [unwired: 1 in, 3 out]
          }
          frame "Lumbares" {
            n751 = Unbundle By Name(w1491) -> ("Lumbares"=w1486:i32)
            n752 = Greater Than 0?(x=w1486) -> (x > 0?=w1488:bool)
            n753 = Subtract(x=w1486, y=5) -> (x-y=w1489:i32)
            n754 = Select(t=w1489, s=w1488, f=w1486) -> (s? t:f=w1487:i32)
            n755 = Bundle By Name(cluster=w1491, "Lumbares"=w1487, "Label"="Lumbares") -> (w1482:T2)
            n756 = Enqueue Element At Opposite End(queue=w1484, element=w1482, error in (no error)=w1483) -> ()  [unwired: 1 in, 3 out]
          }
          frame "Dorsales" {
            n757 = Unbundle By Name(w1501) -> ("Dorsales"=w1496:i32)
            n758 = Greater Than 0?(x=w1496) -> (x > 0?=w1498:bool)
            n759 = Subtract(x=w1496, y=5) -> (x-y=w1499:i32)
            n760 = Select(t=w1499, s=w1498, f=w1496) -> (s? t:f=w1497:i32)
            n761 = Bundle By Name(cluster=w1501, "Dorsales"=w1497, "Label"="Dorsales") -> (w1492:T2)
            n762 = Enqueue Element At Opposite End(queue=w1493, element=w1492, error in (no error)=w1494) -> ()  [unwired: 1 in, 3 out]
          }
          frame "Trapecio" {
            n763 = Unbundle By Name(w1511) -> ("Trapecio"=w1506:i32)
            n764 = Greater Than 0?(x=w1506) -> (x > 0?=w1508:bool)
            n765 = Subtract(x=w1506, y=5) -> (x-y=w1509:i32)
            n766 = Select(t=w1509, s=w1508, f=w1506) -> (s? t:f=w1507:i32)
            n767 = Bundle By Name(cluster=w1511, "Trapecio"=w1507, "Label"="Trapecio") -> (w1503:T2)
            n768 = Enqueue Element At Opposite End(queue=w1505, element=w1503, error in (no error)=w1504) -> ()  [unwired: 1 in, 3 out]
          }
          frame "Pectorales" {
            n769 = Unbundle By Name(w1521) -> ("Pectorales"=w1516:i32)
            n770 = Greater Than 0?(x=w1516) -> (x > 0?=w1518:bool)
            n771 = Subtract(x=w1516, y=5) -> (x-y=w1519:i32)
            n772 = Select(t=w1519, s=w1518, f=w1516) -> (s? t:f=w1517:i32)
            n773 = Bundle By Name(cluster=w1521, "Pectorales"=w1517, "Label"="Pectorales") -> (w1512:T2)
            n774 = Enqueue Element At Opposite End(queue=w1513, element=w1512, error in (no error)=w1514) -> ()  [unwired: 1 in, 3 out]
          }
          frame "Biceps" {
            n775 = Unbundle By Name(w1531) -> ("Biceps"=w1526:i32)
            n776 = Greater Than 0?(x=w1526) -> (x > 0?=w1528:bool)
            n777 = Subtract(x=w1526, y=5) -> (x-y=w1529:i32)
            n778 = Select(t=w1529, s=w1528, f=w1526) -> (s? t:f=w1527:i32)
            n779 = Bundle By Name(cluster=w1531, "Biceps"=w1527, "Label"="Biceps") -> (w1522:T2)
            n780 = Enqueue Element At Opposite End(queue=w1524, element=w1522, error in (no error)=w1523) -> ()  [unwired: 1 in, 3 out]
          }
          frame "Opcional" {
            n781 = Unbundle By Name(w1541) -> ("Opcional"=w1536:i32)
            n782 = Greater Than 0?(x=w1536) -> (x > 0?=w1538:bool)
            n783 = Subtract(x=w1536, y=5) -> (x-y=w1539:i32)
            n784 = Select(t=w1539, s=w1538, f=w1536) -> (s? t:f=w1537:i32)
            n785 = Bundle By Name(cluster=w1541, "Opcional"=w1537, "Label"="Opcional") -> (w1532:T2)
            n786 = Enqueue Element At Opposite End(queue=w1534, element=w1532, error in (no error)=w1533) -> ()  [unwired: 1 in, 3 out]
          }
          frame "Master" {
            n787 = Unbundle By Name(w1551) -> ("Master"=w1546:i32)
            n788 = Greater Than 0?(x=w1546) -> (x > 0?=w1548:bool)
            n789 = Subtract(x=w1546, y=5) -> (x-y=w1549:i32)
            n790 = Select(t=w1549, s=w1548, f=w1546) -> (s? t:f=w1547:i32)
            n791 = Bundle By Name(cluster=w1551, "Master"=w1547, "Label"="Master") -> (w1542:T2)
            n792 = Enqueue Element At Opposite End(queue=w1544, element=w1542, error in (no error)=w1543) -> ()  [unwired: 1 in, 3 out]
          }
          frame Default {
          }
        }
      }
      event "Slider": Value Change {
        n793 = event-data() -> ()  [unwired: 1 in, 6 out]
        n794 = Unbundle By Name(w1557) -> ("Label"=w1555:string)
        n795 = case shown="\"Cuadriceps\"" w1555 {
          tunnel: [w1559 w1565 w1571 w1577 w1583 w1589 w1595 w1601 w1607 w1613 w1619 w1626] -> w1558
          tunnel: w1557 -> [w1564 w1570 w1576 w1582 w1588 w1594 w1600 w1606 w1612 w1618 w1624 w1627]
          tunnel: "Slider" -> [w1563 w1569 w1575 w1581 w1587 w1593 w1599 w1605 w1611 w1617 w1623 w1625]
          tunnel: w1554 -> [w1560 w1567 w1573 w1579 w1584 w1591 w1597 w1603 w1609 w1615 w1621 _]
          tunnel: w1553 -> [w1561 w1566 w1572 w1578 w1585 w1590 w1596 w1602 w1608 w1614 w1620 _]
          frame "Cuadriceps" {
            n796 = Bundle By Name(cluster=w1564, "Cuadriceps"=w1563, "Label"="Cuadriceps") -> (w1559:T2)
            n797 = Enqueue Element At Opposite End(queue=w1561, element=w1559, error in (no error)=w1560) -> ()  [unwired: 1 in, 3 out]
          }
          frame "Isquiotibiales" {
            n798 = Bundle By Name(cluster=w1570, "Isquiotibiales"=w1569, "Label"="Isquiotibiales") -> (w1565:T2)
            n799 = Enqueue Element At Opposite End(queue=w1566, element=w1565, error in (no error)=w1567) -> ()  [unwired: 1 in, 3 out]
          }
          frame "Gluteos" {
            n800 = Bundle By Name(cluster=w1576, "Gluteos"=w1575, "Label"="Gluteos") -> (w1571:T2)
            n801 = Enqueue Element At Opposite End(queue=w1572, element=w1571, error in (no error)=w1573) -> ()  [unwired: 1 in, 3 out]
          }
          frame "Abdomen" {
            n802 = Bundle By Name(cluster=w1582, "Abdomen"=w1581, "Label"="Abdomen") -> (w1577:T2)
            n803 = Enqueue Element At Opposite End(queue=w1578, element=w1577, error in (no error)=w1579) -> ()  [unwired: 1 in, 3 out]
          }
          frame "Lumbares" {
            n804 = Bundle By Name(cluster=w1588, "Lumbares"=w1587, "Label"="Lumbares") -> (w1583:T2)
            n805 = Enqueue Element At Opposite End(queue=w1585, element=w1583, error in (no error)=w1584) -> ()  [unwired: 1 in, 3 out]
          }
          frame "Dorsales" {
            n806 = Bundle By Name(cluster=w1594, "Dorsales"=w1593, "Label"="Dorsales") -> (w1589:T2)
            n807 = Enqueue Element At Opposite End(queue=w1590, element=w1589, error in (no error)=w1591) -> ()  [unwired: 1 in, 3 out]
          }
          frame "Trapecio" {
            n808 = Bundle By Name(cluster=w1600, "Trapecio"=w1599, "Label"="Trapecio") -> (w1595:T2)
            n809 = Enqueue Element At Opposite End(queue=w1596, element=w1595, error in (no error)=w1597) -> ()  [unwired: 1 in, 3 out]
          }
          frame "Pectorales" {
            n810 = Bundle By Name(cluster=w1606, "Pectorales"=w1605, "Label"="Pectorales") -> (w1601:T2)
            n811 = Enqueue Element At Opposite End(queue=w1602, element=w1601, error in (no error)=w1603) -> ()  [unwired: 1 in, 3 out]
          }
          frame "Biceps" {
            n812 = Bundle By Name(cluster=w1612, "Biceps"=w1611, "Label"="Biceps") -> (w1607:T2)
            n813 = Enqueue Element At Opposite End(queue=w1608, element=w1607, error in (no error)=w1609) -> ()  [unwired: 1 in, 3 out]
          }
          frame "Opcional" {
            n814 = Bundle By Name(cluster=w1618, "Opcional"=w1617, "Label"="Opcional") -> (w1613:T2)
            n815 = Enqueue Element At Opposite End(queue=w1614, element=w1613, error in (no error)=w1615) -> ()  [unwired: 1 in, 3 out]
          }
          frame "Master" {
            n816 = Bundle By Name(cluster=w1624, "Master"=w1623, "Label"="Master") -> (w1619:T2)
            n817 = Enqueue Element At Opposite End(queue=w1620, element=w1619, error in (no error)=w1621) -> ()  [unwired: 1 in, 3 out]
          }
          frame "Inicio", Default {
            n818 = Bundle By Name(cluster=w1627, "Slider"=w1625) -> (w1626:T2)
          }
        }
      }
      event "Back": Value Change {
        n819 = event-data() -> ()  [unwired: 1 in, 6 out]
        n820 = Bundle By Name(cluster=w1630, "Label"="Back" ("Message")) -> (w1628:T2)
      }
      event "Master": Value Change {
        n821 = event-data() -> ()  [unwired: 1 in, 6 out]
        n822 = property on="Master" class="Bool (strict)"() -> ("Colors [4]"=w1638:cluster{u32, u32}[])  [unwired: 2 in, 2 out]
        n823 = Index Array(array=w1638) -> (element=w1639:cluster{u32, u32})  [unwired: 1 in]
        n824 = Unbundle(w1639) -> (w1636:u32, w1635:u32)
        n825 = case shown="True" "Master" {
          tunnel: [u32 16448250 ("Boolean Text.Text Colors:Text Color") u32 0 ("Boolean Text.Text Colors:Text Color")] -> w1640
          tunnel: w1636 -> [w1646 w1655]
          tunnel: w1635 -> [_ _]
          tunnel: w1638 -> [w1650 w1657]
          tunnel: [w1647 w1658] -> w1637
          tunnel: w1633 -> [w1644 w1653]
          tunnel: [w1643 w1652] -> w1632
          frame False {
            n826 = Bundle(w1646, "Boolean Text.Text Colors:Text Color"=u32 40709) -> (w1649:T3)  [unwired: 1 in]
            n827 = Bundle By Name(cluster=w1644, "Label"="Inicio") -> (w1643:T2)
            n828 = Replace Array Subset(array=w1650, new element=w1649, index=0) -> (w1647:cluster{u32, u32}[])
          }
          frame True {
            n829 = Bundle(w1655, "Boolean Text.Text Colors:Text Color"=u32 16711680) -> (w1660:T3)  [unwired: 1 in]
            n830 = Bundle By Name(cluster=w1653, "Label"="Master" ("Message")) -> (w1652:T2)
            n831 = Replace Array Subset(array=w1657, new element=w1660, index=0) -> (w1658:cluster{u32, u32}[])
          }
        }
        n832 = property on="Master" class="Bool (strict)"("BoolText.TextColor"=w1640) -> ()  [unwired: 2 in, 2 out]
        n833 = property on="Master" class="Bool (strict)"("Colors [4]"=w1637) -> ()  [unwired: 2 in, 2 out]
        "Master?" <- "Master"
      }
      event "Help": Value Change {
        n834 = event-data() -> ()  [unwired: 1 in, 6 out]
        n835 = call "Help.vi"() -> ()  [unwired: 11 in, 1 out]
      }
      event "Impulso": Value Change {
        n836 = event-data() -> ()  [unwired: 1 in, 6 out]
        n837 = Unbundle By Name(w1671) -> ("Tiempo"=w1669:i32, "Impulso"=w1670:i32, "Ruptura"=w1668:i32, "Frecuencia"=w1667:i32, "Profundidad"=w1666:i32, "Ganancia"=w1665:i32)
        n838 = Build Array(w1669, w1670, w1668, w1667, w1666, w1665) -> (w1664:i32[])
        n839 = call "Impulso.vi"("appended array"=w1664) -> ("Parametros"=w1692:cluster{i32, i32, i32, i32, i32, dbl})  [unwired: 1 in]
        n840 = Unbundle(w1692) -> (w1675:i32, w1673:i32, w1674:i32, w1685:i32, w1679:i32, w1682:dbl)
        n841 = Bundle By Name(cluster=w1671, "Label"="Frecuencia" ("Message"), "Frecuencia"=w1685) -> (w1684:T2)
        n842 = Enqueue Element(queue=w1691, element=w1684, error in (no error)=w1690) -> (queue out=w1688:refnum<queue>, error out=w1689:errorcluster)  [unwired: 1 in, 1 out]
        n843 = Bundle By Name(cluster=w1684, "Label"="Ganancia", "Ganancia"=w1682) -> (w1681:T2)
        n844 = Enqueue Element(queue=w1688, element=w1681, error in (no error)=w1689) -> (queue out=w1686:refnum<queue>, error out=w1687:errorcluster)  [unwired: 1 in, 1 out]
        n845 = Bundle By Name(cluster=w1681, "Label"="Impulso", "Profundidad"=w1679) -> (w1677:T2)
        n846 = Enqueue Element(queue=w1686, element=w1677, error in (no error)=w1687) -> (error out=w1678:errorcluster)  [unwired: 1 in, 2 out]
        n847 = Bundle By Name(cluster=w1677, "Label"="Inicio", "Tiempo"=w1675, "Ruptura"=w1674, "Impulso"=w1673) -> (w1676:T2)
      }
      event "Reset": Value Change {
        n848 = event-data() -> ()  [unwired: 1 in, 6 out]
        n849 = Bundle By Name(cluster=w1744, "Label"="Cuadriceps" ("Message"), "Cuadriceps"=0) -> (w1737:T2)
        n850 = Enqueue Element At Opposite End(queue=w1743, element=w1737, error in (no error)=w1742) -> (queue out=w1740:refnum<queue>, error out=w1741:errorcluster)  [unwired: 1 in, 1 out]
        n851 = Bundle By Name(cluster=w1737, "Label"="Isquiotibiales", "Isquiotibiales"=0) -> (w1735:T2)
        n852 = Enqueue Element At Opposite End(queue=w1740, element=w1735, error in (no error)=w1741) -> (queue out=w1738:refnum<queue>, error out=w1739:errorcluster)  [unwired: 1 in, 1 out]
        n853 = Bundle By Name(cluster=w1735, "Label"="Gluteos", "Gluteos"=0) -> (w1726:T2)
        n854 = Enqueue Element At Opposite End(queue=w1738, element=w1726, error in (no error)=w1739) -> (queue out=w1729:refnum<queue>, error out=w1730:errorcluster)  [unwired: 1 in, 1 out]
        n855 = Bundle By Name(cluster=w1726, "Label"="Abdomen", "Abdomen"=0) -> (w1723:T2)
        n856 = Enqueue Element At Opposite End(queue=w1729, element=w1723, error in (no error)=w1730) -> (queue out=w1727:refnum<queue>, error out=w1728:errorcluster)  [unwired: 1 in, 1 out]
        n857 = Bundle By Name(cluster=w1723, "Label"="Lumbares", "Lumbares"=0) -> (w1720:T2)
        n858 = Enqueue Element At Opposite End(queue=w1727, element=w1720, error in (no error)=w1728) -> (queue out=w1716:refnum<queue>, error out=w1717:errorcluster)  [unwired: 1 in, 1 out]
        n859 = Bundle By Name(cluster=w1720, "Label"="Dorsales", "Dorsales"=0) -> (w1713:T2)
        n860 = Bundle By Name(cluster=w1713, "Label"="Trapecio", "Trapecio"=0) -> (w1710:T2)
        n861 = Enqueue Element At Opposite End(queue=w1716, element=w1713, error in (no error)=w1717) -> (queue out=w1714:refnum<queue>, error out=w1715:errorcluster)  [unwired: 1 in, 1 out]
        n862 = Enqueue Element At Opposite End(queue=w1714, element=w1710, error in (no error)=w1715) -> (queue out=w1707:refnum<queue>, error out=w1706:errorcluster)  [unwired: 1 in, 1 out]
        n863 = Bundle By Name(cluster=w1710, "Label"="Pectorales", "Pectorales"=0) -> (w1705:T2)
        n864 = Bundle By Name(cluster=w1705, "Label"="Biceps", "Biceps"=0) -> (w1700:T2)
        n865 = Enqueue Element At Opposite End(queue=w1707, element=w1705, error in (no error)=w1706) -> (queue out=w1701:refnum<queue>, error out=w1702:errorcluster)  [unwired: 1 in, 1 out]
        n866 = Enqueue Element At Opposite End(queue=w1701, element=w1700, error in (no error)=w1702) -> (queue out=w1696:refnum<queue>, error out=w1697:errorcluster)  [unwired: 1 in, 1 out]
        n867 = Bundle By Name(cluster=w1700, "Label"="Opcional", "Opcional"=0) -> (w1695:T2)
        n868 = Enqueue Element At Opposite End(queue=w1696, element=w1695, error in (no error)=w1697) -> ()  [unwired: 1 in, 3 out]
      }
      event "Start": Value Change {
        n869 = event-data() -> ()  [unwired: 1 in, 6 out]
        n870 = Bundle By Name(cluster=w1753, "Label"="Start" ("Message")) -> (w1752:T2)
        n871 = case shown="True" "Start" {
          tunnel: w1749 -> [w1757 _]
          tunnel: w1748 -> [w1756 w1758]
          tunnel: [w1755 w1758] -> w1747
          frame False {
            n872 = Flush Queue(queue=w1757, error in (no error)=w1756) -> (error out=w1755:errorcluster)  [unwired: 2 out]
          }
          frame True {
          }
        }
        "Start?" <- "Start"
      }
    }
    "Cluster" <- w910
  }
  n873 = Release Queue(queue=w8, error in (no error)=w2) -> ()  [unwired: 1 in, 3 out]
  n874 = VISA Close(VISA resource name=w5, error in (no error)=w4) -> (error out=→"error out 2":errorcluster)
  "error out" <- "error in (no error)"
